vi "MultiQ_09_DataSwitchTimingChanges.vi"() -> ()   [LabVIEW 2021]
doc: "I. Description:\nThis example demonstrates how to acquire a finite amount of data (waveform) using the DAQ device's internal clock.\n\nII. Instructions for Running:\n1. Select the physical channel to correspond to where your signal is input on the DAQ device.\n2. Enter the minimum and maximum voltages.\nNote: For better accuracy try to match the input range to the expected voltage level of the measured signal.\n3. Select the number of samples to acquire.\n4. Set the rate of the acquisition\nNote: The rate should be AT LEAST twice as fast as the maximum frequency component of the signal being acquired.\n\nIII. Block Diagram Steps:\n Steps: \n1. Create an empty task.\n2. Create an analog input voltage channel. Use the DAQmx Base configuration Utility (Tools Menu) to determine the DAQ device name. \n3. Set the rate for the sample clock. Additionally, define the sample mode to be finite and set the number of samples to be acquired per channel.\n4. Call the Start VI to start the acquisition.\n5. Use the Read VI to measure multiple samples from N Channels on the device. Set a timeout so an error is returned if the samples are not returned in the specified time limit\n6. Stop the Analog Input Task.\n7. Call the Clear Task VI to clear the Task.\n8. Use the popup dialog box to display an error if any.\n \nIV. I/O Connections Overview:\nMake sure your signal input terminal matches the Physical Channel I/O Control. For further connection information, refer to your hardware reference manual."
uses:
  <vilib>/Utility/error.llb/DialogType.ctl
  <vilib>/DAQmx/write.llb/DAQmx Write (Analog 2D DBL NChan NSamp).vi
  <vilib>/DAQmx/read.llb/DAQmx Read (Analog 2D DBL NChan NSamp).vi
  <vilib>/measure/maspectr.llb/FFT Power Spectrum and PSD for 1 Chan.vi
  <vilib>/DAQmx/create/channels.llb/DAQmx Create Channel (AI-Voltage-Basic).vi
  <vilib>/DAQmx/configure/timing.llb/DAQmx Timing (Sample Clock).vi
  <vilib>/DAQmx/create/channels.llb/DAQmx Create Channel (AO-Voltage-Basic).vi
  <vilib>/DAQmx/configure/trigger.llb/DAQmx Start Trigger (Digital Edge).vi
  <vilib>/DAQmx/miscellaneous.llb/DAQmx Fill In Error Info.vi
  <vilib>/Analysis/2dsp.llb/Decimate (continuous, DBL).vi
  <vilib>/measure/macond.llb/IIR Filter for 1 Chan.vi
  <vilib>/measure/NI_MAPro.lvlib
  <vilib>/measure/NI_MABase.lvlib
  <vilib>/Analysis/NI_AALPro.lvlib
  <resource>/objmgr/daqmx.rc
panel:
  in  "Run Duration (s) 2":u32=100 caption="Duration (s)"
  out "Nodal Modes":dbl[](array[numeric])=[1092.3, 1649.9, 2505.8]
  out "PlotLabelSize":i32[](array[numeric])
  out "PlotModeSize":i32[](array[numeric])
  out "PlotFreqArray":dbl[][](array[numeric])
  out "PlotLabelArray":string[][](array[string])
  out "Shear Modes":dbl[](array[numeric])=[1092.3, 1649.9, 2505.8]
  out "All Modes":dbl[](array[numeric])=[1092.3, 1649.9, 2505.8]
  out "Modes 10-12":dbl[](array[numeric])=[10072.0, 11259.0, 12454.0]
  out "Modes 7-9":dbl[](array[numeric])=[6683.3, 7225.3, 9346.1]
  in  "Sample Modes":u16(ring)=1 items=["All Modes", "Shear Modes"]
  out "Plot7Label":string="Mode 15: 15961 Hz"
  out "Plot5Label":string="Mode 9: 9346 Hz"
  out "Plot3Label":string="Mode 5: 4361 Hz"
  out "Plot1Label":string="Mode 1: 1092 Hz"
  out "Plot8Label":string="Mode 18: 19859 Hz"
  out "Plot6Label":string="Mode 12: 12454 Hz"
  out "Plot4Label":string="Mode 6: 6645 Hz"
  out "Plot2Label":string="Mode 3: 2506 Hz"
  in  "Ring":u16(ring) items=["EXCITE", "ACQUIRE", "X-Y"]
  in  "Max Value":dbl=10.0 format="%#_13g"
  in  "Min Value":dbl=-10.0 format="%#_13g"
  out "Modes 4-6":dbl[](array[numeric])=[3847.7, 4361.2, 6645.1]
  out "Modes 1-3":dbl[](array[numeric])=[1092.3, 1649.9, 2505.8]
  out "Converted Data Size":i32[](array[numeric])
  out "Raw Data Size":i32[](array[numeric])
  in  "Input Data Type":u16(ring) items=["X Y SUM", "Q 1+/- -- 4+/-", "Q 1-4"]
  in  "Mode Scale":dbl=1.0 min=0.5 max=2.0
  in  "Range (%)":dbl=1.0
  in  "Pressure (t)":sgl=1e-06
  in  "LeverArm (m)":dbl=1.0 min=1.0 max=10000.0
  in  "ADC Range":u16(ring)=6 items=["±0.1 V", "±0.2 V", "±0.5 V", "±1 V", "±2 V", "±5 V", "±10 V"]
  out "PlotLimit":u64
  out "Plot":i32
  in  "Type":u16(ring)=1 items=["Power Spectrum", "PS Density"]
  in  "Unit":u16(ring)=3 items=["Volts", "mRad (full)", "mRad (o2)", "mRad (o1)"]
  in  "Averaging":T1={"Averaging"=enum."No averaging", "weighting mode"=enum."Linear", "number of averages"=10} {"number of averages" min=1 step=1}
  out "Progress":u8(slide) scale=0.0..100.0
  in  "Who":string(combo)="SP"
  in  "fMinPlot":dbl=0.5
  in  "fMaxPlot":dbl=15.0 min=1.0 max=100.0
  in  "Substrate":u16(ring)=1 items=["Silica: 75 x 0.3 mm", "Silica: 75 x 1.0 mm", "Silica: 75 x 2.54 mm"]
  in  "Oversample":bool=TRUE
  in  "fOversample":dbl=50.0 format="%#_13g"
  in  "Span":u32(ring)=60 items=["20 s"=20, "40 s"=40, "1 min"=60, "3 min"=180, "5 min"=300]
  in  "Offset (V)":sgl=2.0
  in  "Ampl. (V)":sgl=2.0
  out "NAve":dbl format="%#_13g"
  out "ADCScale":dbl format="%#_13g"
  out "SizeTimeSeries":i32
  out "BufferPeriod":dbl format="%#_13g"
  out "PSD X":cluster{"f0":dbl, "df":dbl, dbl[][]}(graph)
  out "PlotUnitIndex":u16
  out "DataFilePath":path
  out "fSampleAcquire":dbl format="%#_13g"
  out "NDataPointsOutput":u64
  out "DeltaTOutput":dbl format="%#_13g"
  out "fSampleOutput":dbl format="%#_13g"
  out "DecimFactor":u32
  in  "Comment":string
  out "WriteNumber":i32
  out "WriteLimit":i32
  out "Step":i32
  out "Location":string
  out "PathAtOpen":path
  out "PathAtClose":path
  out "RunLight":bool
  in  "Temp Path":path
  in  "stop":bool
  out "Plot8":cluster{"f0":dbl, "df":dbl, dbl[][]}(graph)
  out "Plot7":cluster{"f0":dbl, "df":dbl, dbl[][]}(graph)
  out "WriteNewHeader":bool
  out "TempFilePath":path
  out "RunPeriod":dbl format="%#_13g"
  out "NDataPointsAcquire":u64
  out "nPlotPerRun":u64
  out "InitialArray":dbl[][](array[numeric])
  out "time vector":dbl[](array[numeric])
  out "ReZero":dbl[][](array[numeric])
  out "df":dbl format="%#_13g"
  out "PlotPeriod":dbl format="%#_13g"
  in  "Run Duration (s)":u32=100 caption="Duration (s)"
  in  "Run Number":i8=1
  in  "∆f (Hz)":u32(ring)=1 items=["1.00"=1, "0.50"=2, "0.25"=4, "0.10"=10]
  in  "Excite":bool
  out "# Elements Response Queue":i32
  out "BufferPeriod ms":u32
  out "# Elements Drive Queue":i32
  out "High Pass IIR filter specs":T2={"Topology"=enum."Butterworth", "Type"=enum."Bandpass", "Order"=7, "Lower Fc"=2000.0, "Upper Fc"=3800.0, "PB Ripple"=0.025, "SB Attenuation"=90.0}
  out "DeltaTAcquire":dbl format="%#_13g"
  out "BufferPoints":u32
  out "PlotPoints":u32
  out "nBufferPerPlot":u32
  out "fMaxPlotHz":dbl format="%#_13g"
  out "fMinPlotHz":dbl format="%#_13g"
  out "Plot6":cluster{"f0":dbl, "df":dbl, dbl[][]}(graph)
  out "Plot5":cluster{"f0":dbl, "df":dbl, dbl[][]}(graph)
  out "Plot4":cluster{"f0":dbl, "df":dbl, dbl[][]}(graph)
  out "Plot3":cluster{"f0":dbl, "df":dbl, dbl[][]}(graph)
  out "Plot2":cluster{"f0":dbl, "df":dbl, dbl[][]}(graph)
  out "Plot1":cluster{"f0":dbl, "df":dbl, dbl[][]}(graph)
  in  "Start":bool
  out "PSD Y":cluster{"f0":dbl, "df":dbl, dbl[][]}(graph) caption="Measurement"
  out "File":string
  in  "Path":path caption="File Name"
  in  "Label":string
  in  "Name":string
  out "HTML \nTitle":string
  out "Start Time":timestamp
  out "Write Light":bool
  in  "AutoSave":bool=TRUE
  in  "Manual Save":bool=TRUE caption="Saving Data"
  out "Out":path caption="File Name Out"
  in  "QUIT":bool
  # "Acquire"
  # "Multi Q\nVer 0.9.5.0 • July 2021\nSteve Penn"
  # "Sample"
  # "Comment"
  # "Frequency"
  # "kHz"
  # ":"
  # "Oversample"
  # "kHz"
  # "PLOT:"
  # "Mode Plots:"
  # "PSD Y / Excitation"
  # "/"
  # "Averaging"
  # "Drive"
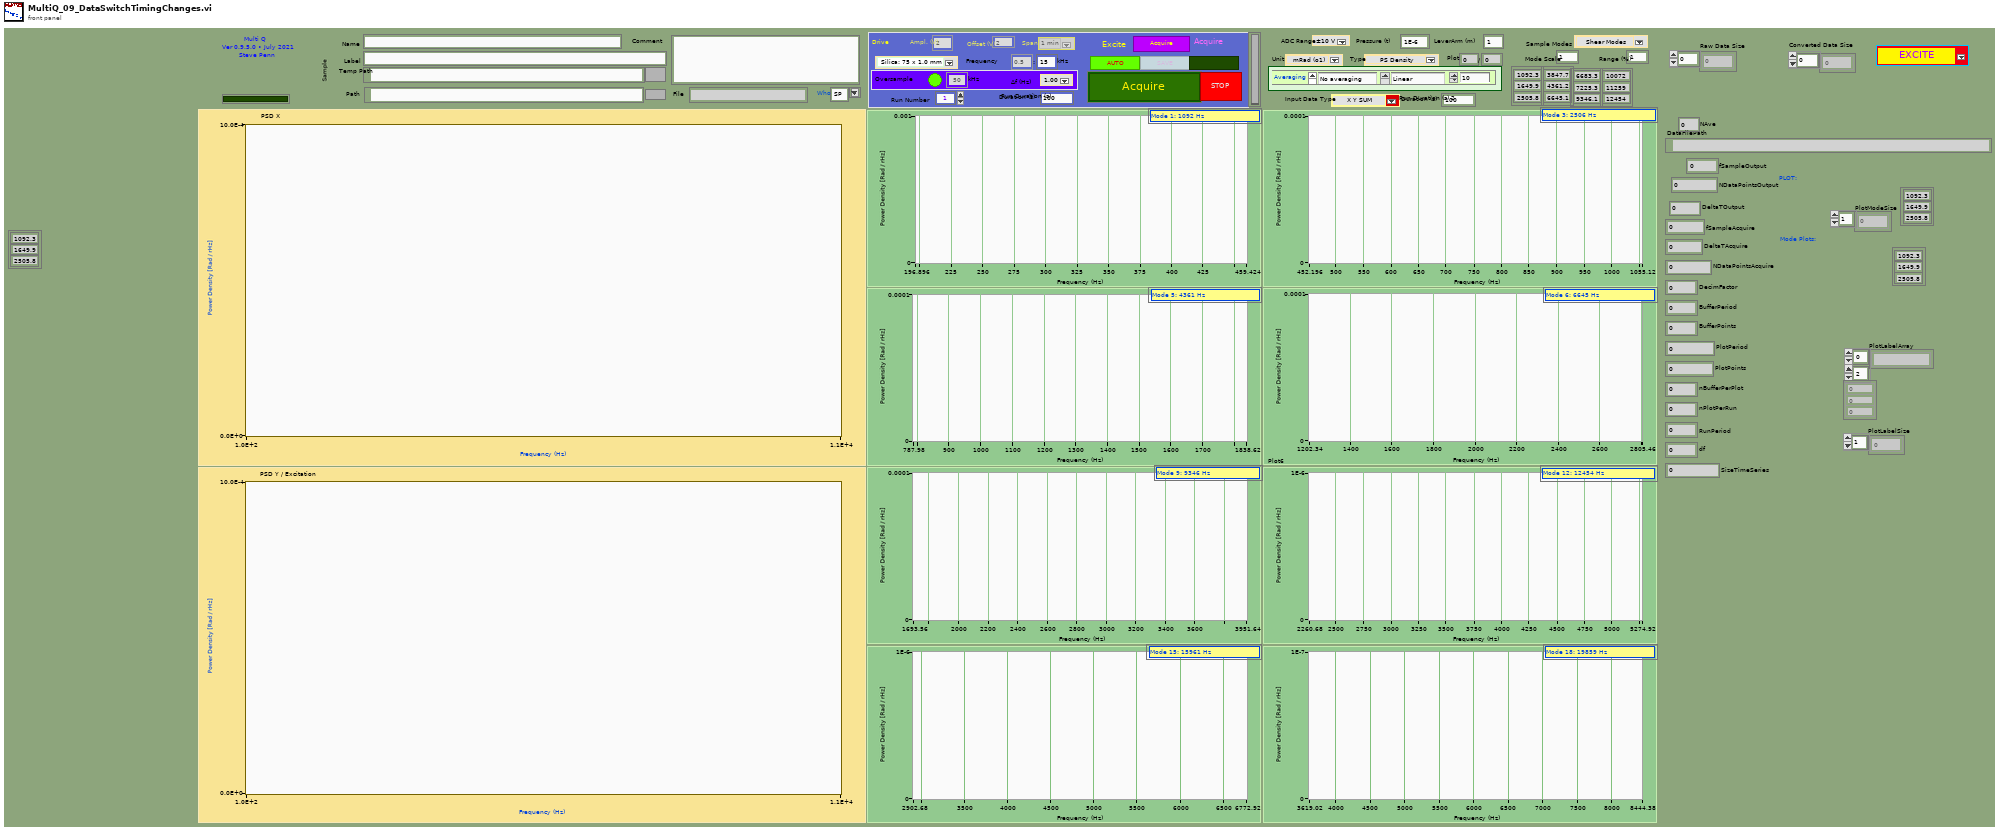
[diagram p1: front panel]
types:
  T1 = cluster{"Averaging":enum16{"No averaging", "Vector averaging", "RMS averaging", "Peak hold"}, "weighting mode":enum16{"Linear", "Exponential"}, "number of averages":u32}
  T2 = cluster{"Topology":enum16{"Off", "Butterworth", "Chebyshev", "Inverse Chebyshev", "Elliptic", "Bessel"}, "Type":enum16{"Lowpass", "Highpass", "Bandpass", "Bandstop"}, "Order":i32, "Lower Fc":dbl, "Upper Fc":dbl, "PB Ripple":dbl, "SB Attenuation":dbl}
  T3 = enum16{"Off", "Butterworth", "Chebyshev", "Inverse Chebyshev", "Elliptic", "Bessel"}
  T4 = enum16{"Lowpass", "Highpass", "Bandpass", "Bandstop"}
  T5 = enum8{"open", "replace", "create", "open or create", "replace or create", "replace or create with confirmation"}
  T6 = enum16{"No averaging", "Vector averaging", "RMS averaging", "Peak hold"}
  T7 = cluster{"Averaging":enum16{"No averaging", "Vector averaging", "RMS averaging", "Peak hold"}, "weighting mode":enum16{"Linear", "Exponential"}, "weighting mode":u64}
  T8 = typedef "DialogType.ctl" = u16
  T9 = enum16{"Left Button", "Center Button", "Right Button", "Window Close"}
  T10 = cluster{"Averaging":enum16{"No averaging", "Vector averaging", "RMS averaging", "Peak hold"}, "weighting mode":enum16{"Linear", "Exponential"}, "Value":u64}
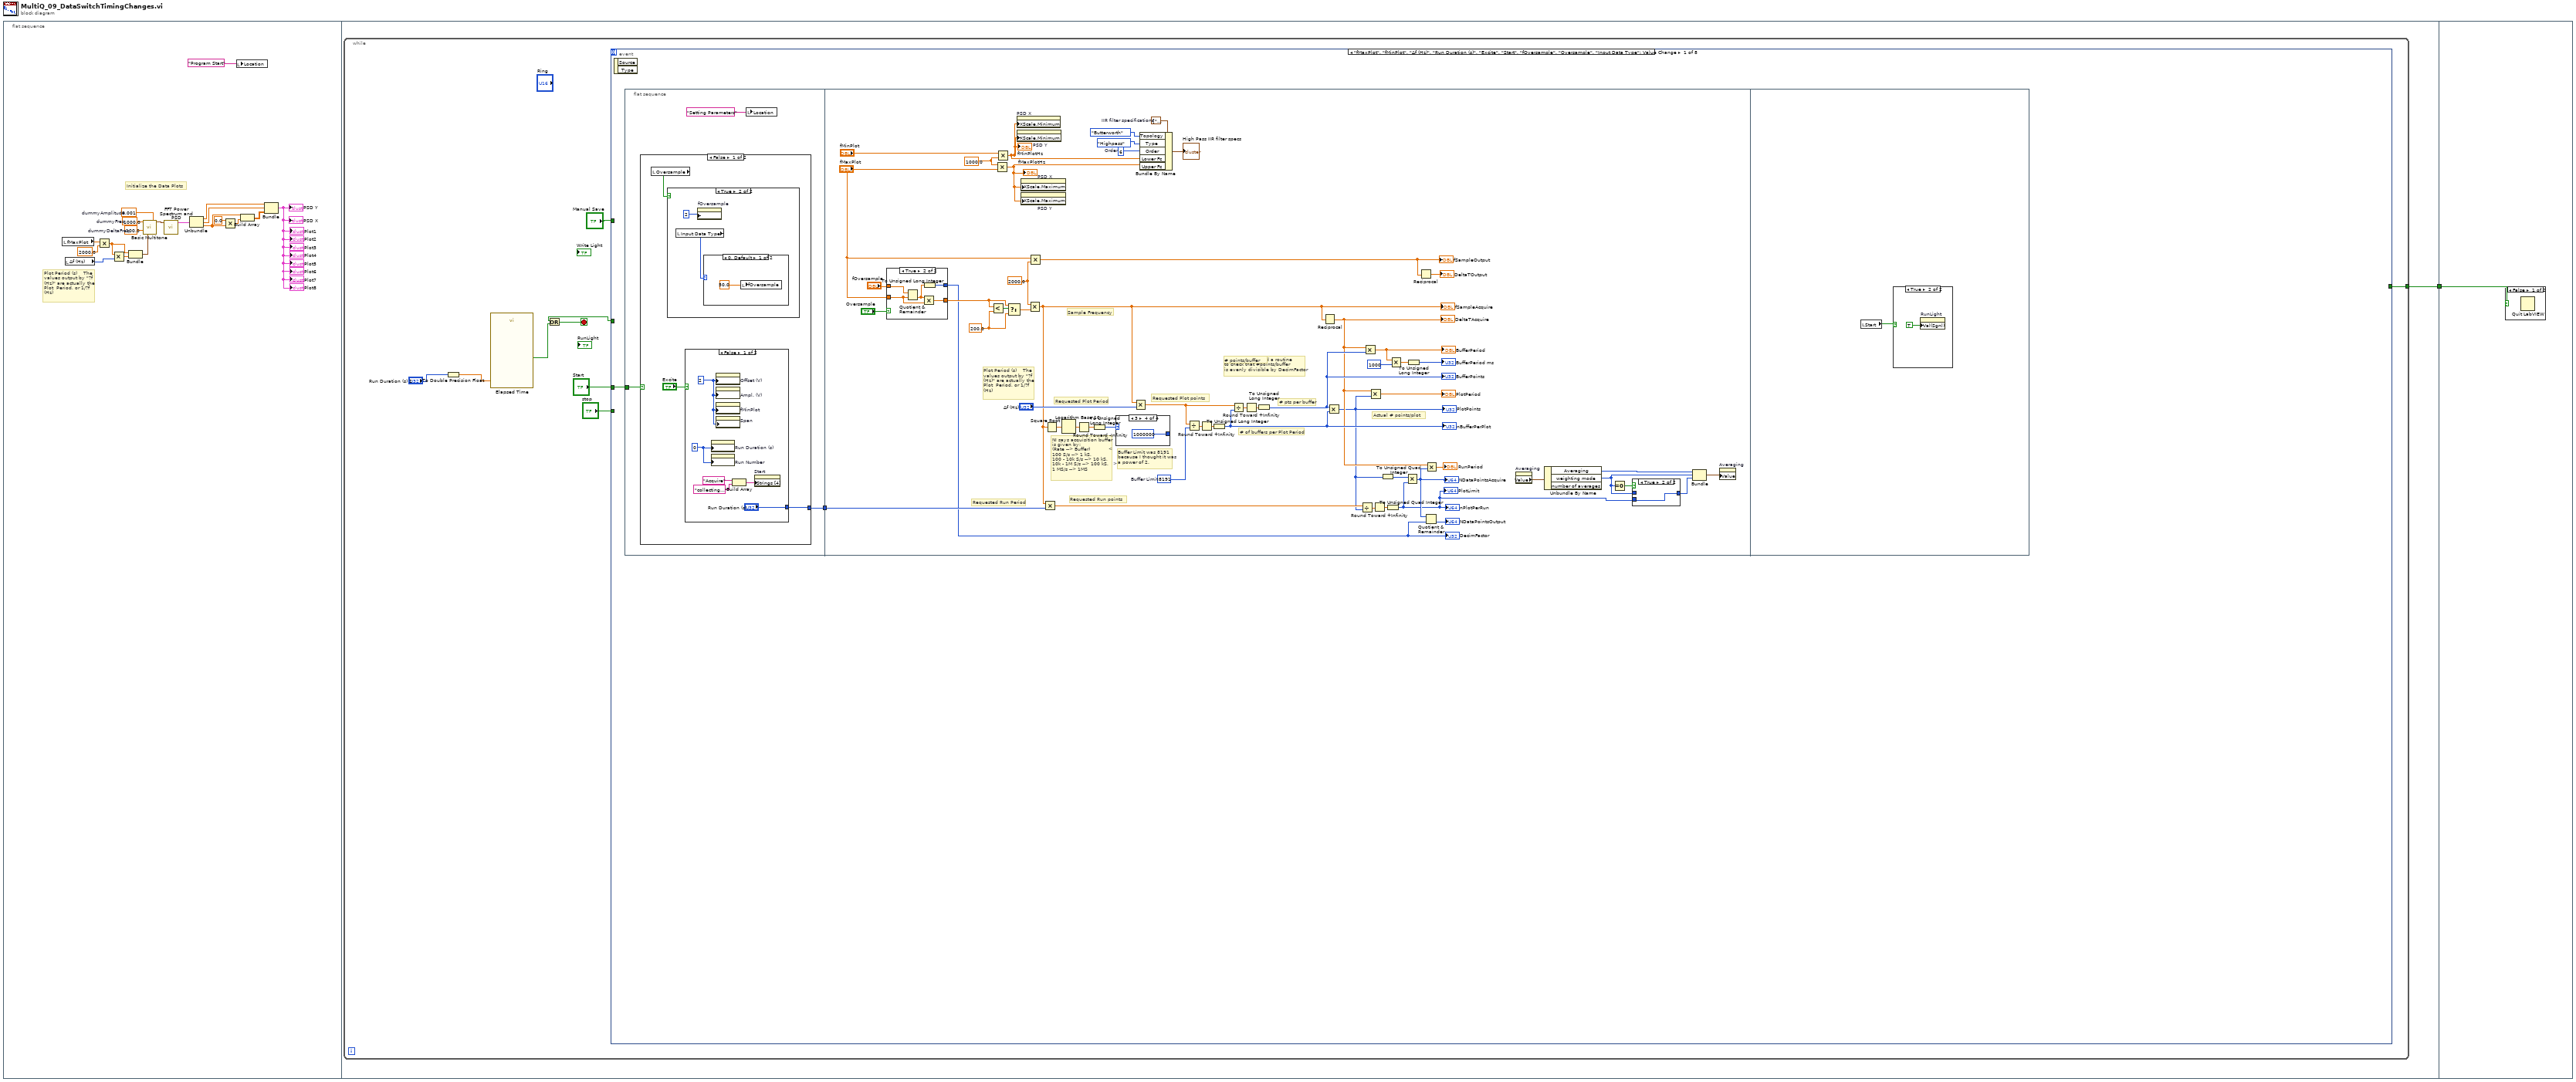
[diagram p0: block diagram]
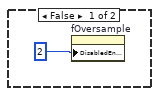
[diagram p2: hidden frame]
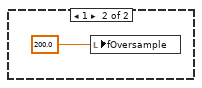
[diagram p3: hidden frame]
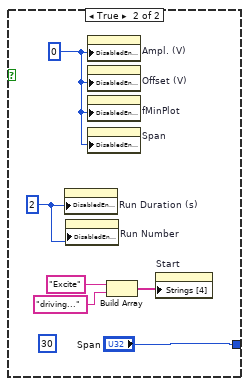
[diagram p4: hidden frame]
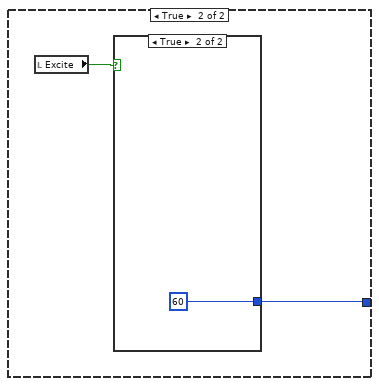
[diagram p5: hidden frame]
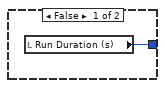
[diagram p6: hidden frame]
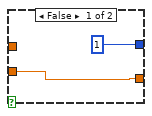
[diagram p8: hidden frame]
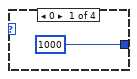
[diagram p9: hidden frame]
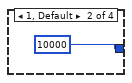
[diagram p10: hidden frame]
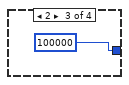
[diagram p11: hidden frame]
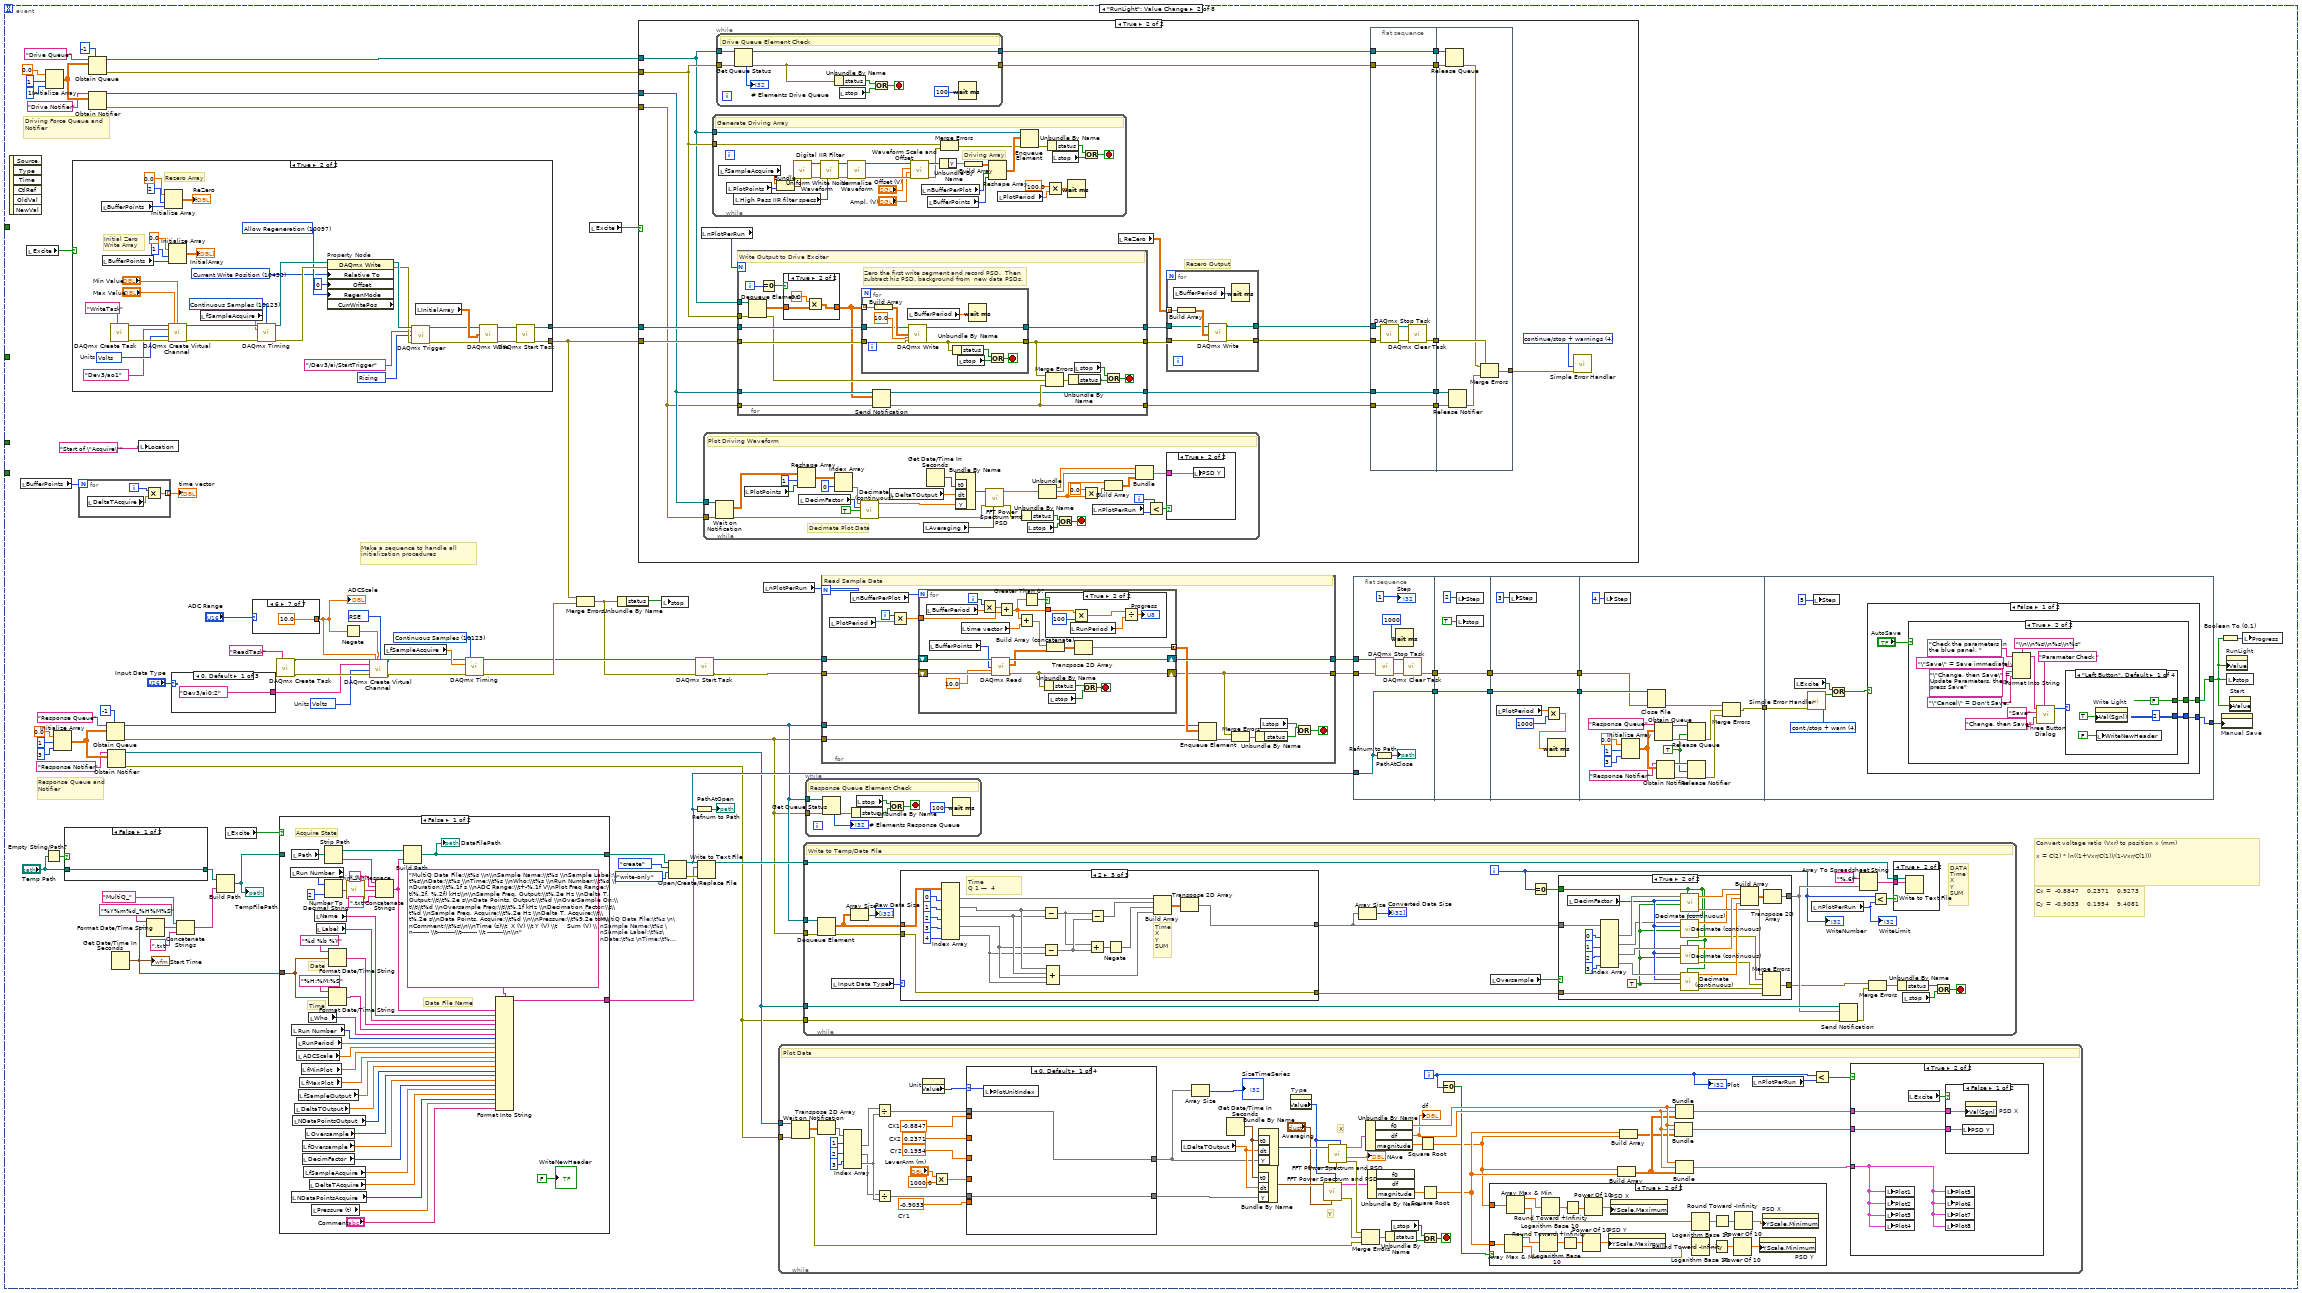
[diagram p13: hidden frame]
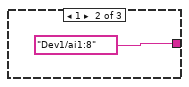
[diagram p14: hidden frame]
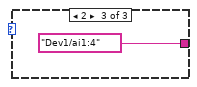
[diagram p15: hidden frame]
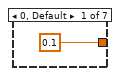
[diagram p16: hidden frame]
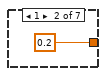
[diagram p17: hidden frame]
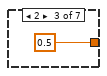
[diagram p18: hidden frame]
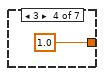
[diagram p19: hidden frame]
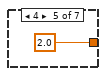
[diagram p20: hidden frame]
diagram:
  n1 = flat-sequence {
    tunnel: [w21] -> w1
    tunnel: w1 -> [w1123]
    frame #0 {
      w4 = 0.001  # dummyAmplitude
      w2 = 100.0  # dummyDeltaFreq
      w3 = 1000.0  # dummyFreq
      # "Initialize the Data Plots"
      # "Plot Period (s)    The values output by \"?f (Hz)\" are actually the Plot  Period, or 1/?f (Hz)"
      n2 = local read "fMaxPlot"() -> (w9:dbl)
      n3 = local read "∆f (Hz)"() -> (w8:u32)
      n4 = Multiply(x=w9, y=2000.0) -> (x*y=w6:dbl)
      n5 = Multiply(x=w6, y=w8) -> (x*y=w7:dbl)
      n6 = Bundle(w6, w7) -> (w19:cluster{dbl, dbl})  [unwired: 1 in]
      n7 = call <vilib>:"Basic Multitone.vi"("start frequency"=w3, "amplitude"=w4, "delta frequency"=w2, "sampling info"=w19) -> ("signal out"=w18:waveform(dbl))  [unwired: 8 in, 3 out]
      n8 = call-poly <vilib>:"FFT Power Spectrum and PSD.vi"("time signal"=w18) -> ("Power Spectrum / PSD"=w11:cluster{"f0":dbl, "df":dbl, "magnitude":dbl[]})  [unwired: 7 in, 3 out]
      n9 = Unbundle(w11) -> ("f0"=w16:dbl, "df"=w13:dbl, "magnitude"=w12:dbl[])
      n10 = Multiply(x=0.0, y=w12) -> (x*y=w14:dbl[])
      n11 = local write "Location"("Program Start") -> ()
      n12 = Build Array(w12, w14) -> (w15:dbl[][])
      n13 = Bundle("f0"=w16, "df"=w13, w15) -> (→"PSD Y" →"PSD X" →"Plot5" →"Plot6" →"Plot7" →"Plot8" →"Plot3" →"Plot1" →"Plot2" →"Plot4":cluster{"f0":dbl, "df":dbl, dbl[][]})  [unwired: 1 in]
    }
    frame #1 {
      n14 = while {
        tunnel: [w30] -> w21
        stop <- w22 stop-if-true
        n15 = To Double Precision Float(number="Run Duration (s) 2") -> (double precision float=w25:dbl)
        n16 = call "Elapsed Time"("Time Target (s)"=w25) -> ("Time has Elapsed"=w24:bool)  [unwired: 11 in, 7 out]
        n17 = event shown="[0] \"fMaxPlot\", \"fMinPlot\", \"∆f (Hz)\", \"Run Duration (s)\", \"Excite\", \"Start\", \"fOversample\", \"Oversample\", \"Input Data Type\": Value Change" {
          selector: _ -> [_ _ _ _ _ _ _ _]
          dyn-events: _ -> [_ _ _ _ _ _ _ _]
          timeout: _ -> [_ _ _ _ _ _ _ _]
          tunnel: [_ _ _ _ _ _ w1098 _] -> w23
          tunnel: [_ _ _ _ _ _ w1099 _] -> w30
          tunnel: "Manual Save" -> [_ _ _ _ _ _ _ _]
          tunnel: "Start" -> [w31 _ _ _ _ _ _ _]
          tunnel: "stop" -> [_ _ _ _ _ _ _ _]
          event "fMaxPlot", "fMinPlot", "∆f (Hz)", "Run Duration (s)", "Excite", "Start", "fOversample", "Oversample", "Input Data Type": Value Change {
            n18 = event-data() -> ()  [unwired: 3 out]
            n19 = flat-sequence {
              tunnel: [w35] -> w32
              tunnel: w31 -> [w34]
              tunnel: w32 -> [w81]
              frame #0 {
                n20 = case shown="False" w34 {
                  tunnel: [w37 w56] -> w35
                  frame False {
                    n21 = local read "Oversample"() -> (w36:bool)
                    n22 = case shown="True" w36 {
                      frame False {
                        n23 = property on="fOversample" class="DigNum (strict)"("DisabledEnum"=2) -> ()  [unwired: 2 in, 2 out]
                      }
                      frame True {
                        n24 = local read "Input Data Type"() -> (w40:u16)
                        n25 = property on="fOversample" class="DigNum (strict)"("DisabledEnum"=2) -> ()  [unwired: 2 in, 2 out]
                        n26 = case shown="0, Default" w40 {
                          frame 0, Default {
                            n27 = local write "fOversample"(50.0) -> ()
                          }
                          frame 1 {
                            n28 = local write "fOversample"(200.0) -> ()
                          }
                        }
                      }
                    }
                    n29 = case shown="False" "Excite" {
                      tunnel: ["Run Duration (s)" "Span"] -> w37
                      frame False {
                        w46 = 0
                        w44 = 2
                        n30 = property on="Run Duration (s)" class="DigNum (strict)"("DisabledEnum"=w46) -> ()  [unwired: 2 in, 2 out]
                        n31 = property on="Run Number" class="DigNum (strict)"("DisabledEnum"=w46) -> ()  [unwired: 2 in, 2 out]
                        n32 = property on="Offset (V)" class="DigNum (strict)"("DisabledEnum"=w44) -> ()  [unwired: 2 in, 2 out]
                        n33 = property on="Ampl. (V)" class="DigNum (strict)"("DisabledEnum"=w44) -> ()  [unwired: 2 in, 2 out]
                        n34 = property on="fMinPlot" class="DigNum (strict)"("DisabledEnum"=w44) -> ()  [unwired: 2 in, 2 out]
                        n35 = property on="Span" class="Ring (strict)"("DisabledEnum"=w44) -> ()  [unwired: 2 in, 2 out]
                        n36 = Build Array("Acquire", "collecting...") -> (w49:string[])
                        n37 = property on="Start" class="Bool (strict)"("Strings [4]"=w49) -> ()  [unwired: 2 in, 2 out]
                      }
                      frame True {
                        (unwired) 30
                        w52 = 2
                        w51 = 0
                        n38 = property on="Run Duration (s)" class="DigNum (strict)"("DisabledEnum"=w52) -> ()  [unwired: 2 in, 2 out]
                        n39 = property on="Run Number" class="DigNum (strict)"("DisabledEnum"=w52) -> ()  [unwired: 2 in, 2 out]
                        n40 = property on="Ampl. (V)" class="DigNum (strict)"("DisabledEnum"=w51) -> ()  [unwired: 2 in, 2 out]
                        n41 = property on="Offset (V)" class="DigNum (strict)"("DisabledEnum"=w51) -> ()  [unwired: 2 in, 2 out]
                        n42 = property on="fMinPlot" class="DigNum (strict)"("DisabledEnum"=w51) -> ()  [unwired: 2 in, 2 out]
                        n43 = property on="Span" class="Ring (strict)"("DisabledEnum"=w51) -> ()  [unwired: 2 in, 2 out]
                        n44 = Build Array("Excite", "driving...") -> (w55:string[])
                        n45 = property on="Start" class="Bool (strict)"("Strings [4]"=w55) -> ()  [unwired: 2 in, 2 out]
                      }
                    }
                  }
                  frame True {
                    n46 = local read "Excite"() -> (w57:bool)
                    n47 = case shown="True" w57 {
                      tunnel: [w58 60] -> w56
                      frame False {
                        n48 = local read "Run Duration (s)"() -> (w58:u32)
                      }
                      frame True {
                      }
                    }
                  }
                }
                n49 = local write "Location"("Setting Parameters") -> ()
              }
              frame #1 {
                w102 = 6  # Order
                w105 = T2 {"Topology"=enum."Butterworth", "Type"=enum."Bandpass", "Order"=7, "Lower Fc"=2000.0, "Upper Fc"=3800.0, "PB Ripple"=0.025, "SB Attenuation"=90.0}  # IIR filter specifications
                w111 = 1000.0
                w91 = 8191  # Buffer Limit
                w78 = 2000.0
                w110 = 200.0
                # "# pts per buffer"
                # "I may need to add a routine \nto check that #points/buffer\nis evenly divisible by DecimFactor"
                # "Requested Run points"
                # "Requested Run Period"
                # "Requested Plot Period"
                # "NI says acquisition buffer  is given by:                   (Rate --> Buffer)            < 100 S/s --> 1 kS,                 100 - 10k S/s --> 10 kS,   10k - 1M S/s --> 100 kS,   > 1 MS/s --> 1MS"
                # "Buffer Limit was 8191 because I thought it was a power of 2."
                # "Plot Period (s)    The values output by \"?f (Hz)\" are actually the Plot  Period, or 1/?f (Hz)"
                # "Sample Frequency"
                # "Actual # points/plot"
                # "# points/buffer"
                # "Requested Plot points"
                # "# of buffers per Plot Period"
                n50 = case shown="True" "Oversample" {
                  tunnel: "fOversample" -> [_ w124]
                  tunnel: [w119 w123] -> w79
                  tunnel: "fMaxPlot" -> [w119 w122]
                  tunnel: [1 w121] -> w71
                  frame False {
                  }
                  frame True {
                    n51 = Quotient & Remainder(x=w124, y=w122) -> (floor(x/y)=w120:dbl)  [unwired: 1 out]
                    n52 = Multiply(x=w120, y=w122) -> (x*y=w123:dbl)
                    n53 = To Unsigned Long Integer(number=w120) -> (unsigned 32bit integer=w121:u32)
                  }
                }
                "DecimFactor" <- w71
                n54 = Less?(x=w79, y=w110) -> (x < y?=w115:bool)
                n55 = Multiply(x=w111, y="fMaxPlot") -> (x*y=w69:dbl)
                "fMaxPlotHz" <- w69
                n56 = Multiply(x="fMinPlot", y=w111) -> (x*y=w70:dbl)
                "fMinPlotHz" <- w70
                n57 = Select(t=w79, s=w115, f=w110) -> (s? t:f=w114:dbl)
                n58 = property on="PSD X" class="WFGraph (strict)"("XScale.Minimum"=w70) -> ()  [unwired: 2 in, 2 out]
                n59 = property on="PSD Y" class="WFGraph (strict)"("XScale.Minimum"=w70) -> ()  [unwired: 2 in, 2 out]
                n60 = property on="PSD X" class="WFGraph (strict)"("XScale.Maximum"=w69) -> ()  [unwired: 2 in, 2 out]
                n61 = property on="PSD Y" class="WFGraph (strict)"("XScale.Maximum"=w69) -> ()  [unwired: 2 in, 2 out]
                n62 = Multiply(x=w78, y=w114) -> (x*y=w88:dbl)
                "fSampleAcquire" <- w88
                n63 = Multiply(x="fMaxPlot", y=w78) -> (x*y=w76:dbl)
                "fSampleOutput" <- w76
                n64 = Multiply(x=w88, y=w81) -> (x*y=w87:dbl)
                n65 = Square Root(x=w88) -> (sqrt(x)=w96:dbl)
                n66 = Logarithm Base 10(1:w96) -> (0:w95:dbl)
                n67 = Round Toward -Infinity(1:w95) -> (0:w94:dbl)
                n68 = To Unsigned Long Integer(number=w94) -> (unsigned 32bit integer=w93:u32)
                n69 = case shown="3" w93 {
                  tunnel: [1000 10000 100000 1000000] -> _
                  frame 0 {
                  }
                  frame 1, Default {
                  }
                  frame 2 {
                  }
                  frame 3 {
                  }
                }
                n70 = Multiply(x=w88, y="∆f (Hz)") -> (x*y=w113:dbl)
                n71 = Bundle By Name(cluster=w105, "Topology"=T3."Butterworth", "Type"=T4."Highpass" ("Enum"), "Order"=w102, "Lower Fc"=w70, "Upper Fc"=w69) -> (→"High Pass IIR filter specs":T2)
                n72 = Divide(x=w113, y=w91) -> (x/y=w109:dbl)
                n73 = Round Toward +Infinity(x=w109) -> (ceil(x): smallest int >= x=w108:dbl)
                n74 = To Unsigned Long Integer(number=w108) -> (unsigned 32bit integer=w106:u32)
                "nBufferPerPlot" <- w106
                n75 = Divide(x=w113, y=w106) -> (x/y=w112:dbl)
                n76 = Round Toward +Infinity(x=w112) -> (ceil(x): smallest int >= x=w107:dbl)
                n77 = To Unsigned Long Integer(number=w107) -> (unsigned 32bit integer=w84:u32)
                "BufferPoints" <- w84
                n78 = Reciprocal(x=w88) -> (1/x=w83:dbl)
                "DeltaTAcquire" <- w83
                n79 = Multiply(x=w84, y=w106) -> (x*y=w60:u32)
                "PlotPoints" <- w60
                n80 = Divide(x=w87, y=w60) -> (x/y=w86:dbl)
                n81 = Multiply(x=w83, y=w84) -> (x*y=w99:dbl)
                "BufferPeriod" <- w99
                n82 = Multiply(x=w83, y=w60) -> (x*y=→"PlotPeriod":dbl)
                n83 = Round Toward +Infinity(x=w86) -> (ceil(x): smallest int >= x=w85:dbl)
                n84 = To Unsigned Quad Integer(1:w60) -> (0:w61:u64)
                n85 = To Unsigned Quad Integer(1:w85) -> (0:w62:u64)
                "nPlotPerRun" <- w62
                "PlotLimit" <- w62
                n86 = Multiply(x=w99, y=1000) -> (x*y=w98:dbl)
                n87 = Multiply(x=w61, y=w62) -> (x*y=w74:u64)
                "NDataPointsAcquire" <- w74
                n88 = To Unsigned Long Integer(number=w98) -> (unsigned 32bit integer=→"BufferPeriod ms":u32)
                n89 = Reciprocal(x=w76) -> (1/x=→"DeltaTOutput":dbl)
                n90 = Quotient & Remainder(x=w74, y=w71) -> (floor(x/y)=→"NDataPointsOutput":u64)  [unwired: 1 out]
                n91 = Multiply(x=w83, y=w74) -> (x*y=→"RunPeriod":dbl)
                n92 = property on="Averaging" class="Clust (strict)"() -> ("Value"=w64:T1)  [unwired: 2 in, 2 out]
                n93 = Unbundle By Name(w64) -> ("Averaging"=w65:T6, "weighting mode"=w68:enum16{"Linear", "Exponential"})  [unwired: 1 out]
                n94 = Equal To 0?(x=w68) -> (x = 0?=w66:bool)
                n95 = case shown="True" w66 {
                  tunnel: [w116 w117] -> w67
                  tunnel: w68 -> [w116 _]
                  tunnel: w62 -> [_ w117]
                  frame False {
                  }
                  frame True {
                  }
                }
                n96 = Bundle("Averaging"=w65, "weighting mode"=w68, "weighting mode"=w67) -> (w63:T7)  [unwired: 1 in]
                n97 = property on="Averaging" class="Clust (strict)"("Value"=w63) -> ()  [unwired: 2 in, 2 out]
              }
              frame #2 {
                n98 = local read "Start"() -> (w129:bool)
                n99 = case shown="True" w129 {
                  frame False {
                  }
                  frame True {
                    n100 = property on="RunLight" class="Bool (strict)"("Val(Sgnl)"=TRUE) -> ()  [unwired: 2 in, 2 out]
                  }
                }
              }
            }
          }
          event "RunLight": Value Change {
            w139 = 10123 items=["Finite Samples"=10178, "Continuous Samples"=10123] ("sample mode")
            w141 = 10348 items=["Volts"=10348]  # Units
            w146 = 10083 items=["default"=-1, "differential"=10106, "RSE"=10083, "NRSE"=10078] ("input terminal configuration")
            # "Cx =  -0.8847    0.2371    0.9273\n\nCy =  -0.9033    0.1954    9.4081"
            # "Convert voltage ratio (Vxr) to position x (mm)\n\nx = C(2) * ln((1+Vxr/C(1))/(1-Vxr/C(1)))"
            # "Response Queue and Notifier"
            # "Driving Force Queue and Notifier"
            # "Make a sequence to handle all initialization procedures"
            n101 = event-data() -> ()  [unwired: 7 out]
            n102 = local read "BufferPoints"() -> (w202:u32)
            n103 = local read "Excite"() -> (w199:bool)
            n104 = Empty String/Path?(string/path="Temp Path") -> (empty?=w187:bool)
            n105 = Initialize Array(0.0, 1, 1) -> (w176:dbl[][])
            n106 = Initialize Array(0.0, 1, 3) -> (w165:dbl[][])
            n107 = case shown="False" w187 {
              tunnel: "Temp Path" -> [w480 _]
              tunnel: [w480 w481] -> w185
              frame False {
              }
              frame True {
                w481 = path "/Users/qlab/Documents/MultiQ/Temp"
                n108 = local write "Temp Path"(w481) -> ()
              }
            }
            n109 = case shown="True" w199 {
              tunnel: [w687 w694] -> w198
              tunnel: [w688 w695] -> w200
              frame False {
                n110 = call <vilib>:"DAQmx Create Task.vi"() -> ("task out"=w688:refnum<k21>, "error out"=w687:errorcluster)  [unwired: 14 in]
              }
              frame True {
                w690 = 10430 items=["First Sample"=10424, "Current Write Position"=10430] ("RelativeTo")
                w703 = 10097 items=["Allow Regeneration"=10097, "Do Not Allow Regeneration"=10158] ("RegenMode")
                w699 = 10280 items=["Falling"=10171, "Rising"=10280]
                w706 = 10123 items=["Finite Samples"=10178, "Continuous Samples"=10123] ("sample mode")
                w710 = 10348 items=["Volts"=10348]  # Units
                # "Initial Zero Write Array"
                # "Rezero Array"
                n111 = local read "BufferPoints"() -> (w721:u32)
                n112 = local read "BufferPoints"() -> (w719:u32)
                n113 = call <vilib>:"DAQmx Create Task.vi"("new task name"="WriteTask") -> ("task out"=w712:refnum<k21>, "error out"=w711:errorcluster)  [unwired: 13 in]
                n114 = Initialize Array(0.0, 2, w721) -> (→"ReZero":dbl[][])
                n115 = Initialize Array(0.0, 1, w719) -> (→"InitialArray":dbl[][])
                n116 = call-poly <vilib>:"DAQmx Create Virtual Channel.vi"("task in"=w712, "maximum value"="Max Value", "minimum value"="Min Value", "physical channels"=tag "Dev3/ao1", "units"=w710, "error in"=w711) -> ("task out"=w709:refnum<k21>, "error out"=w708:errorcluster)  [unwired: 8 in]
                n117 = local read "fSampleAcquire"() -> (w707:dbl)
                n118 = call-poly <vilib>:"DAQmx Timing.vi"("task/channels in"=w709, "sample mode"=w706, "rate"=w707, "error in"=w708) -> ("task out"=w705:refnum<k21>, "error out"=w704:errorcluster)  [unwired: 10 in]
                n119 = property on="Property Node" class="DAQmx Write" props=["Relative To", "Offset", "RegenMode", "CurrWritePos"](reference=w705, error in=w704, "Relative To"=w690, "Offset"=0, "RegenMode"=w703) -> (reference out=w702:refnum<k21>, error out=w701:errorcluster)  [unwired: 1 out]
                n120 = call-poly <vilib>:"DAQmx Trigger.vi"("task/channels in"=w702, "source"=tag "/Dev3/ai/StartTrigger" ("DAQmx Terminal"), "edge"=w699, "error in"=w701) -> ("task out"=w697:refnum<k21>, "error out"=w696:errorcluster)  [unwired: 10 in]
                n121 = local read "InitialArray"() -> (w698:dbl[][])
                n122 = call-poly <vilib>:"DAQmx Write.vi"("task/channels in"=w697, "data"=w698, "error in"=w696) -> ("task out"=w692:refnum<k21>, "error out"=w693:errorcluster)  [unwired: 10 in, 1 out]
                n123 = call <vilib>:"DAQmx Start Task.vi"("task/channels in"=w692, "error in"=w693) -> ("task out"=w695:refnum<k21>, "error out"=w694:errorcluster)  [unwired: 12 in]
              }
            }
            n124 = for {
              N: w202 -> [_]
              tunnel: [w811] -> w201 mode=indexing
              i -> [w809]
              n125 = local read "DeltaTAcquire"() -> (w810:dbl)
              n126 = Multiply(x=w809, y=w810) -> (x*y=w811:dbl)
            }
            "time vector" <- w201
            n127 = Obtain Queue(max queue size (-1, unlimited)=-1, name (unnamed)="Drive Queue", element data type=w176) -> (queue out=w167:refnum<queue>, error out=w166:errorcluster)  [unwired: 2 in, 1 out]
            n128 = Obtain Notifier(name (unnamed)="Drive Notifier", notification data type=w176) -> (notifier out=w169:refnum<notifier>, error out=w168:errorcluster)  [unwired: 2 in, 1 out]
            n129 = Obtain Queue(max queue size (-1, unlimited)=-1, name (unnamed)="Response Queue", element data type=w165) -> (queue out=w157:refnum<queue>, error out=w156:errorcluster)  [unwired: 2 in, 1 out]
            n130 = Obtain Notifier(name (unnamed)="Response Notifier", notification data type=w165) -> (notifier out=w155:refnum<notifier>, error out=w154:errorcluster)  [unwired: 2 in, 1 out]
            n131 = Get Date/Time In Seconds() -> (seconds since 1Jan1904=w184:timestamp)
            "Start Time" <- w184
            n132 = local write "Location"("Start of \"Acquire\"") -> ()
            n133 = Format Date/Time String(time format string (%c)="%Y%m%d_%H%M%S", seconds (now)=w184) -> (date/time string=w210:string)  [unwired: 1 in]
            n134 = case shown="0, Default" "Input Data Type" {
              tunnel: [tag "Dev3/ai0:2" ("DAQmx Physical Channel") tag "Dev1/ai1:8" ("DAQmx Physical Channel") tag "Dev1/ai1:4" ("DAQmx Physical Channel")] -> w140
              frame 0, Default {
              }
              frame 1 {
              }
              frame 2 {
              }
            }
            n135 = Concatenate Strings("MultiQ_", w210, ".txt") -> (w189:string)
            n136 = Build Path(base path=w185, name or relative path=w189) -> (appended path=w188:path)
            "TempFilePath" <- w188
            n137 = local read "Excite"() -> (w196:bool)
            n138 = case shown="6" "ADC Range" {
              tunnel: [0.1 ("Max Value") 0.2 ("Max Value") 0.5 ("Max Value") 1.0 ("Max Value") 2.0 ("Max Value") 5.0 ("Max Value") 10.0 ("Max Value")] -> w145
              frame 0, Default {
              }
              frame 1 {
              }
              frame 2 {
              }
              frame 3 {
              }
              frame 4 {
              }
              frame 5 {
              }
              frame 6 {
              }
            }
            "ADCScale" <- w145
            n139 = call <vilib>:"DAQmx Create Task.vi"("new task name"="ReadTask") -> ("task out"=w143:refnum<k21>, "error out"=w142:errorcluster)  [unwired: 13 in]
            n140 = case shown="False" w196 {
              tunnel: [w499 w523] -> w205
              tunnel: w184 -> [w508 w522]
              tunnel: [w498 w521] -> w195
              tunnel: w188 -> [_ w521]
              frame False {
                w507 = "MultiQ Data File:\\t%s \\n\\nSample Name:\\t%s \\nSample Label:\\t%s\\nDate:\\t%s \\nTime:\\t%s \\nWho:\\t%s \\nRun Number:\\t%d \\nDuration:\\t%.1f s \\nADC Range:\\t+-%.1f V\\nPlot Freq Range:\\t(%.2f, %.2f) kHz\\n\\nSample Freq, Output:\\t%.2e Hz \\nDelta T, Output:\\t\\t%.2e s\\nData Points, Output:\\t%d \\nOverSample On:\\t\\t\\t%d \\nOversample Freq:\\t\\t%.1f kHz \\nDecimation Factor:\\t\\t%d \\nSample Freq, Acquire:\\t%.2e Hz \\nDelta T, Acquire:\\t\\t%.2e s\\nData Points, Acquire:\\t%d \\n\\nPressure:\\t%9.2e torr\\nComment:\\t%s\\n\\nTime (s)\\t  X (V) \\t Y (V) \\t     Sum (V) \\n-------- \\t---------\\t-------- \\t --------\\n\\n"  # MultiQ Data File:\t%s \n\nSample Name:\t%s \nSample Label:\t%s\nDate:\t%s \nTime:\t%s \nWho:\t%s \nRun Number:\t%d \nDuration:\t%.1f s \nADC Range:\t+-%.1f V\nPlot Freq Range:\t(%.2f, %.2f) kHz\n\nSample Freq, Output:\t%.2e Hz \nDelta T, Output:\t\t%.2e s\nData Points, Output:\t%d \nOverSample On:\t\t\t%d \nOversample Freq:\t\t%.1f kHz \nDecimation Factor:\t\t%d \nSample Freq, Acquire:\t%.2e Hz \nDelta T, Acquire:\t\t%.2e s\nData Points, Acquire:\t%d \n\nPressure:\t%9.2e torr\nComment:\t%s\n\nTime (s)\t  X (V) \t Y (V) \t     Sum (V) \n-------- \t---------\t-------- \t --------\n\n
                # "Data File Name"
                # "Date"
                # "Time"
                # "Acquire State"
                n141 = local read "Run Number"() -> (w512:i8)
                n142 = local read "NDataPointsAcquire"() -> (w484:u64)
                n143 = local read "Path"() -> (w511:path)
                n144 = local read "Run Number"() -> (w506:i8)
                n145 = local read "NDataPointsOutput"() -> (w491:u64)
                n146 = local read "DeltaTOutput"() -> (w490:dbl)
                n147 = local read "RunPeriod"() -> (w500:dbl)
                n148 = local read "ADCScale"() -> (w495:dbl)
                n149 = local read "fSampleOutput"() -> (w492:dbl)
                n150 = local read "fMaxPlot"() -> (w493:dbl)
                n151 = local read "fMinPlot"() -> (w494:dbl)
                n152 = local read "fOversample"() -> (w488:dbl)
                n153 = local read "DecimFactor"() -> (w487:u32)
                n154 = local read "fSampleAcquire"() -> (w486:dbl)
                n155 = local read "Oversample"() -> (w489:bool)
                n156 = local read "Who"() -> (w496:string)
                n157 = local read "DeltaTAcquire"() -> (w485:dbl)
                n158 = local read "Pressure (t)"() -> (w483:sgl)
                n159 = local read "Name"() -> (w502:string)
                n160 = local read "Label"() -> (w503:string)
                n161 = Strip Path(path=w511) -> (stripped path=w517:path, name=w514:string)
                n162 = Number To Decimal String(number=w512, width (-)=2) -> (decimal integer string=w518:string)
                n163 = Format Date/Time String(time format string (%c)="%d %b %Y", seconds (now)=w508) -> (date/time string=w504:string)  [unwired: 1 out]
                n164 = Format Date/Time String(time format string (%c)="%H:%M:%S", seconds (now)=w508) -> (date/time string=w505:string)  [unwired: 1 out]
                n165 = call <vilib>:"Trim Whitespace.vi"("string"=w518) -> ("trimmed string"=w515:string)  [unwired: 1 in]
                n166 = Concatenate Strings(w514, "_", w515, ".txt") -> (w501:string)
                n167 = Build Path(base path=w517, name or relative path=w501) -> (appended path=w498:path)
                "DataFilePath" <- w498
                n168 = Format Into String(format string=w507, w501, w502, w503, w504, w505, w496, w506, w500, w495, w494, w493, w492, w490, w491, w489, w488, w487, w486, w485, w484, w483, "Comment") -> (resulting string=w499:string)  [unwired: 2 in, 1 out]
                "WriteNewHeader" <- FALSE
              }
              frame True {
                # "Exciter State"
                # "Date"
                # "Time"
                n169 = Format Date/Time String(time format string (%c)="%d %b %Y", seconds (now)=w522) -> (date/time string=w525:string)  [unwired: 1 out]
                n170 = Format Date/Time String(time format string (%c)="%H:%M:%S", seconds (now)=w522) -> (date/time string=w524:string)  [unwired: 1 out]
                n171 = local write "WriteNewHeader"(FALSE) -> ()
                n172 = Format Into String(format string="Date:\\t%s \\nTime:\\t %s \\n\\nTime (s)\\t  X (V) \\t Y (V) \\t     Sum (V) \\n-------- \\t---------\\t-------- \\t --------\\n\\n", w525, w524) -> (resulting string=w523:string)  [unwired: 2 in, 1 out]
              }
            }
            n173 = Negate(x=w145) -> (-x=w144:dbl)
            n174 = call-poly <vilib>:"DAQmx Create Virtual Channel.vi"("task in"=w143, "maximum value"=w145, "minimum value"=w144, "input terminal configuration"=w146, "physical channels"=w140, "units"=w141, "error in"=w142) -> ("task out"=w137:refnum<k21>, "error out"=w136:errorcluster)  [unwired: 7 in]
            n175 = local read "fSampleAcquire"() -> (w138:dbl)
            n176 = call-poly <vilib>:"DAQmx Timing.vi"("task/channels in"=w137, "sample mode"=w139, "rate"=w138, "error in"=w136) -> ("task out"=w134:refnum<k21>, "error out"=w135:errorcluster)  [unwired: 10 in]
            n177 = Merge Errors(w198, w135) -> (w133:errorcluster)
            n178 = local read "Excite"() -> (w197:bool)
            n179 = Unbundle By Name(w133) -> ("status"=w190:bool)
            n180 = case shown="True" w197 {
              tunnel: w200 -> [w530 w551]
              tunnel: w198 -> [w529 w550]
              tunnel: w166 -> [w533 w549]
              tunnel: w169 -> [w532 w548]
              tunnel: w168 -> [w531 w547]
              tunnel: w167 -> [w534 w545]
              frame False {
                n181 = Release Queue(queue=w534, error in (no error)=w533) -> ()  [unwired: 1 in, 3 out]
                n182 = Release Notifier(notifier=w532, error in (no error)=w531) -> ()  [unwired: 1 in, 3 out]
                n183 = call <vilib>:"DAQmx Clear Task.vi"("task in"=w530, "error in"=w529) -> ()  [unwired: 13 in, 1 out]
              }
              frame True {
                w546 = T8 4 items=["no dialog", "OK message", "continue or stop message", "OK message + warnings", "continue/stop + warnings"] ("type of dialog (OK msg:1)")
                # "Rezero Output"
                n184 = local read "nPlotPerRun"() -> (w557:u64)
                n185 = while {
                  tunnel: w548 -> [w606]
                  tunnel: w547 -> [w605]
                  i -> [w592]
                  stop <- w594 stop-if-true
                  # "Decimate Plot Data"
                  # "Plot Driving Waveform"
                  n186 = Wait on Notification(notifier=w606, error in (no error)=w605) -> (notification=w604:dbl[][], error out=w583:errorcluster)  [unwired: 2 in, 2 out]
                  n187 = local read "PlotPoints"() -> (w602:u32)
                  n188 = Reshape Array(w604, 1, w602) -> (w601:dbl[][])
                  n189 = local read "DecimFactor"() -> (w589:u32)
                  n190 = Index Array(array=w601, index (row)=0) -> (element=w587:dbl[])  [unwired: 1 in]
                  n191 = call-poly <vilib>:"Decimate (continuous).vi"("error in (no error)"=w583, "averaging"=TRUE, "decimating factor"=w589, "X"=w587) -> ("error out"=w584:errorcluster, "Decimated Array"=w586:dbl[])  [unwired: 6 in]
                  n192 = local read "DeltaTOutput"() -> (w599:dbl)
                  n193 = local read "Averaging"() -> (w585:T1)
                  n194 = Get Date/Time In Seconds() -> (seconds since 1Jan1904=w598:timestamp)
                  n195 = Bundle By Name("t0"=w598, "dt"=w599, "Y"=w586) -> (w597:waveform(dbl))  [unwired: 1 in]
                  n196 = call-poly <vilib>:"FFT Power Spectrum and PSD.vi"("averaging parameters"=w585, "error in (no error)"=w584, "time signal"=w597) -> ("error out"=w596:errorcluster, "Power Spectrum / PSD"=w576:cluster{"f0":dbl, "df":dbl, "magnitude":dbl[]})  [unwired: 5 in, 2 out]
                  n197 = Unbundle By Name(w596) -> ("status"=w595:bool)
                  n198 = local read "stop"() -> (w593:bool)
                  n199 = Unbundle(w576) -> ("f0"=w581:dbl, "df"=w578:dbl, "magnitude"=w577:dbl[])
                  n200 = Or(x=w595, y=w593) -> (x .or. y?=w594:bool)
                  n201 = Multiply(x=0.0, y=w577) -> (x*y=w579:dbl[])
                  n202 = local read "nPlotPerRun"() -> (w591:u64)
                  n203 = Build Array(w577, w579) -> (w580:dbl[][])
                  n204 = Bundle("f0"=w581, "df"=w578, w580) -> (w575:cluster{"f0":dbl, "df":dbl, dbl[][]})  [unwired: 1 in]
                  n205 = Less?(x=w592, y=w591) -> (x < y?=w590:bool)
                  n206 = case shown="True" w590 {
                    tunnel: w575 -> [_ w607]
                    frame False {
                    }
                    frame True {
                      n207 = local write "PSD Y"(w607) -> ()
                    }
                  }
                }
                n208 = while {
                  tunnel: w545 -> [w658]
                  tunnel: w549 -> [w654]
                  stop <- w650 stop-if-true
                  # "Driving Array"
                  # "Generate Driving Array"
                  n209 = local read "fSampleAcquire"() -> (w665:dbl)
                  n210 = local read "PlotPoints"() -> (w664:u32)
                  n211 = local read "High Pass IIR filter specs"() -> (w660:T2)
                  n212 = Bundle("fSampleAcquire"=w665, "PlotPoints"=w664) -> (w666:cluster{"fSampleAcquire":dbl, "PlotPoints":u32})  [unwired: 1 in]
                  n213 = call <vilib>:"Uniform White Noise Waveform.vi"("sampling info"=w666) -> ("error out"=w676:errorcluster, "signal out"=w675:waveform(dbl))  [unwired: 9 in]
                  n214 = call-poly <vilib>:"Digital IIR Filter.vi"("IIR filter specifications"=w660, "error in (no error)"=w676, "signal in"=w675) -> ("error out"=w674:errorcluster, "signal out"=w673:waveform(dbl))  [unwired: 6 in, 1 out]
                  n215 = call <vilib>:"Normalize Waveform.vi"("error in (no error)"=w674, "waveform in"=w673) -> ("error out"=w672:errorcluster, "normalized waveform"=w671:waveform(dbl))  [unwired: 6 in, 2 out]
                  n216 = call <vilib>:"Waveform Scale and Offset.vi"("error in (no error)"=w672, "scale"="Ampl. (V)", "offset"="Offset (V)", "waveform in"=w671) -> ("error out"=w653:errorcluster, "waveform out"=w667:waveform(dbl))  [unwired: 6 in]
                  n217 = local read "nBufferPerPlot"() -> (w663:u32)
                  n218 = local read "BufferPoints"() -> (w662:u32)
                  n219 = Unbundle By Name(w667) -> ("Y"=w668:dbl[])
                  n220 = Merge Errors(w654, w653) -> (w655:errorcluster)
                  n221 = Build Array(w668) -> (w677:dbl[][])
                  n222 = Reshape Array(w677, w663, w662) -> (w661:dbl[][])
                  n223 = local read "PlotPeriod"() -> (w656:dbl)
                  n224 = Enqueue Element(queue=w658, element=w661, error in (no error)=w655) -> (error out=w652:errorcluster)  [unwired: 1 in, 2 out]
                  n225 = Multiply(x=100.0, y=w656) -> (x*y=w659:dbl)
                  n226 = Unbundle By Name(w652) -> ("status"=w651:bool)
                  n227 = local read "stop"() -> (w649:bool)
                  n228 = Wait (ms)(milliseconds to wait=w659) -> ()  [unwired: 1 out]
                  n229 = Or(x=w651, y=w649) -> (x .or. y?=w650:bool)
                }
                n230 = while {
                  tunnel: w545 -> [w684]
                  tunnel: w549 -> [w683]
                  tunnel: [w679] -> w540
                  tunnel: [w678] -> w542
                  stop <- w681 stop-if-true
                  # "Drive Queue Element Check"
                  n231 = Get Queue Status(queue=w684, error in (no error)=w683) -> (queue out=w678:refnum<queue>, error out=w679:errorcluster, # elements in queue=→"# Elements Drive Queue":i32)  [unwired: 1 in, 5 out]
                  n232 = Unbundle By Name(w679) -> ("status"=w682:bool)
                  n233 = local read "stop"() -> (w680:bool)
                  n234 = Or(x=w682, y=w680) -> (x .or. y?=w681:bool)
                  n235 = Wait (ms)(milliseconds to wait=100) -> ()  [unwired: 1 out]
                }
                n236 = for {
                  N: w557 -> [_]
                  tunnel: w545 -> [w629]
                  tunnel: w549 -> [w628]
                  tunnel: w551 -> [w631]
                  tunnel: [w633] -> w555
                  tunnel: w550 -> [w630]
                  tunnel: [w632] -> w556
                  tunnel: w548 -> [w624]
                  tunnel: w547 -> [w623]
                  tunnel: [w622] -> w537
                  tunnel: [w621] -> w535
                  i -> [w618]
                  stop <- w625 stop-if-true
                  # "Zero the first write segment and record PSD.  Then subtract his PSD. background from  new data PSDs."
                  # "Write Output to Drive Exciter"
                  n237 = Dequeue Element(queue=w629, error in (no error)=w628) -> (element=w616:dbl[][], error out=w627:errorcluster)  [unwired: 1 in, 2 out]
                  n238 = Equal To 0?(x=w618) -> (x = 0?=w617:bool)
                  n239 = case shown="True" w617 {
                    tunnel: w616 -> [w634 w637]
                    tunnel: [w634 w635] -> w615
                    frame False {
                    }
                    frame True {
                      n240 = Multiply(x=0.0, y=w637) -> (x*y=w635:dbl[][])
                    }
                  }
                  n241 = for {
                    tunnel: w631 -> [w638]
                    tunnel: w630 -> [w641]
                    tunnel: [w643] -> w633
                    tunnel: [w642] -> w632
                    tunnel: w615 -> [w645] mode=indexing
                    stop <- w647 stop-if-true
                    n242 = Build Array(w645) -> (w639:dbl[][])
                    n243 = local read "BufferPeriod"() -> (w646:dbl)
                    n244 = call-poly <vilib>:"DAQmx Write.vi"("task/channels in"=w638, "data"=w639, "timeout"=10.0, "error in"=w641) -> ("task out"=w643:refnum<k21>, "error out"=w642:errorcluster)  [unwired: 9 in, 1 out]
                    n245 = Unbundle By Name(w642) -> ("status"=w648:bool)
                    n246 = local read "stop"() -> (w644:bool)
                    n247 = Wait (ms)(milliseconds to wait=w646) -> ()  [unwired: 1 out]
                    n248 = Or(x=w648, y=w644) -> (x .or. y?=w647:bool)
                  }
                  n249 = Send Notification(notification=w615, notifier=w624, error in (no error)=w623) -> (notifier out=w621:refnum<notifier>, error out=w622:errorcluster)
                  n250 = Merge Errors(w632, w627, w622) -> (w626:errorcluster)
                  n251 = Unbundle By Name(w626) -> ("status"=w620:bool)
                  n252 = local read "stop"() -> (w619:bool)
                  n253 = Or(x=w619, y=w620) -> (x .or. y?=w625:bool)
                }
                n254 = local read "ReZero"() -> (w554:dbl[][])
                n255 = for {
                  tunnel: w554 -> [w613] mode=indexing
                  tunnel: w556 -> [w612]
                  tunnel: w555 -> [w610]
                  tunnel: [w609] -> w553
                  tunnel: [w608] -> w552
                  n256 = local read "BufferPeriod"() -> (w614:dbl)
                  n257 = Build Array(w613) -> (w611:dbl[][])
                  n258 = call-poly <vilib>:"DAQmx Write.vi"("task/channels in"=w610, "data"=w611, "error in"=w612) -> ("task out"=w609:refnum<k21>, "error out"=w608:errorcluster)  [unwired: 10 in, 1 out]
                  n259 = Wait (ms)(milliseconds to wait=w614) -> ()  [unwired: 1 out]
                }
                n260 = flat-sequence {
                  tunnel: w553 -> [w562]
                  tunnel: w552 -> [w561]
                  tunnel: [w558] -> w543
                  tunnel: w542 -> [w566]
                  tunnel: [w566] -> w541
                  tunnel: w540 -> [w565]
                  tunnel: [w565] -> w539
                  tunnel: [w564] -> w538
                  tunnel: w537 -> [w564]
                  tunnel: [w563] -> w536
                  tunnel: w535 -> [w563]
                  tunnel: [w570] -> w544
                  tunnel: w543 -> [w568]
                  tunnel: w541 -> [w574]
                  tunnel: w539 -> [w573]
                  tunnel: w538 -> [w572]
                  tunnel: w536 -> [w571]
                  frame #0 {
                    n261 = call <vilib>:"DAQmx Stop Task.vi"("task/channels in"=w562, "error in"=w561) -> ("task out"=w560:refnum<k21>, "error out"=w559:errorcluster)  [unwired: 12 in]
                    n262 = call <vilib>:"DAQmx Clear Task.vi"("task in"=w560, "error in"=w559) -> ("error out"=w558:errorcluster)  [unwired: 13 in]
                  }
                  frame #1 {
                    n263 = Release Queue(queue=w574, error in (no error)=w573) -> (error out=w567:errorcluster)  [unwired: 1 in, 2 out]
                    n264 = Release Notifier(notifier=w571, error in (no error)=w572) -> (error out=w569:errorcluster)  [unwired: 1 in, 2 out]
                    n265 = Merge Errors(w567, w568, w569) -> (w570:errorcluster)
                  }
                }
                n266 = call <vilib>:"Simple Error Handler.vi"("type of dialog (OK msg:1)"=w546, "error in (no error)"=w544) -> ()  [unwired: 3 in, 5 out]
              }
            }
            n267 = local write "stop"(w190) -> ()
            n268 = Open/Create/Replace File(file path (use dialog)=w195, operation (0:open)=T5."create", access (0:read/write)=enum16{"read/write", "read-only", "write-only"}."write-only") -> (refnum out=w158:refnum<file>, error out=w208:errorcluster)  [unwired: 1 in, 3 out]
            n269 = call <vilib>:"DAQmx Start Task.vi"("task/channels in"=w134, "error in"=w133) -> ("task out"=w131:refnum<k21>, "error out"=w132:errorcluster)  [unwired: 12 in]
            n270 = Refnum to Path(1:w158) -> (0:→"PathAtOpen":path)
            n271 = Write to Text File(file (use dialog)=w158, text=w205, error in=w208) -> (refnum out=w181:refnum<file>)  [unwired: 3 out]
            n272 = local read "nPlotPerRun"() -> (w203:u64)
            n273 = while {
              tunnel: w155 -> [w366]
              tunnel: w154 -> [w365]
              i -> [w333]
              stop <- w367 stop-if-true
              w347 = -0.9033  # CY1
              w348 = 0.1954  # CY2
              w349 = 0.2371  # CX2
              w350 = -0.8847  # CX1
              # "Y"
              # "X"
              # "Plot Data"
              n274 = Wait on Notification(notifier=w366, error in (no error)=w365) -> (notification=w370:dbl[][], error out=w369:errorcluster)  [unwired: 2 in, 2 out]
              n275 = Transpose 2D Array(2D array=w370) -> (transposed array=w381:dbl[][])
              n276 = Index Array(array=w381, index (row) #1=1, index (row) #2=2, index (row) #3=3) -> (element #1=w376:dbl[], element #2=w374:dbl[], element #3=w375:dbl[])  [unwired: 3 in]
              n277 = Divide(x=w376, y=w375) -> (x/y=w352:dbl[])
              n278 = Divide(x=w374, y=w375) -> (x/y=w353:dbl[])
              n279 = property on="Unit" class="Ring (strict)"() -> ("Value"=w345:u16)  [unwired: 2 in, 2 out]
              n280 = Multiply(x="LeverArm (m)", y=1000.0) -> (x*y=w340:dbl)
              n281 = case shown="0, Default" w345 {
                selector: w345 -> [w402 w405 w431 w457]
                tunnel: w353 -> [w403 w428 w455 w472]
                tunnel: w352 -> [w404 w414 w453 w470]
                tunnel: [w403 w420 w454 w471] -> w351
                tunnel: [w404 w411 w429 w462] -> w338
                tunnel: w350 -> [_ w410 w452 w469]
                tunnel: w349 -> [_ w409 w451 w468]
                tunnel: w348 -> [_ w408 w430 w467]
                tunnel: w340 -> [_ w407 w450 w466]
                tunnel: w347 -> [_ w406 w449 w465]
                frame 0, Default {
                  n282 = local write "PlotUnitIndex"(w402) -> ()
                }
                frame 1 {
                  n283 = Divide(x=w414, y=w410) -> (x/y=w419:dbl[])
                  n284 = Divide(x=w409, y=w407) -> (x/y=w412:dbl)
                  n285 = Divide(x=w408, y=w407) -> (x/y=w421:dbl)
                  n286 = Divide(x=w428, y=w406) -> (x/y=w427:dbl[])
                  n287 = local write "PlotUnitIndex"(w405) -> ()
                  n288 = Increment(x=w419) -> (x+1=w416:dbl[])
                  n289 = Decrement(x=w419) -> (x-1=w418:dbl[])
                  n290 = Increment(x=w427) -> (x+1=w424:dbl[])
                  n291 = Decrement(x=w427) -> (x-1=w426:dbl[])
                  n292 = Negate(x=w418) -> (-x=w417:dbl[])
                  n293 = Negate(x=w426) -> (-x=w425:dbl[])
                  n294 = Divide(x=w424, y=w425) -> (x/y=w423:dbl[])
                  n295 = Divide(x=w416, y=w417) -> (x/y=w415:dbl[])
                  n296 = Natural Logarithm(1:w423) -> (0:w422:dbl[])
                  n297 = Natural Logarithm(1:w415) -> (0:w413:dbl[])
                  n298 = Multiply(x=w413, y=w412) -> (x*y=w411:dbl[])
                  n299 = Multiply(x=w421, y=w422) -> (x*y=w420:dbl[])
                }
                frame 2 {
                  w439 = 2.0
                  n300 = Divide(x=w455, y=w449) -> (x/y=w434:dbl[])
                  n301 = Divide(x=w453, y=w452) -> (x/y=w444:dbl[])
                  n302 = Square(x=w434) -> (x^2=w438:dbl[])
                  n303 = Divide(x=w451, y=w450) -> (x/y=w443:dbl)
                  n304 = Divide(x=w430, y=w450) -> (x/y=w440:dbl)
                  n305 = Square(x=w444) -> (x^2=w448:dbl[])
                  n306 = Divide(x=w438, y=3.0) -> (x/y=w436:dbl[])
                  n307 = Divide(x=w448, y=3.0) -> (x/y=w446:dbl[])
                  n308 = Multiply(x=w443, y=w439) -> (x*y=w442:dbl)
                  n309 = Multiply(x=w439, y=w440) -> (x*y=w432:dbl)
                  n310 = Increment(x=w436) -> (x+1=w435:dbl[])
                  n311 = Increment(x=w446) -> (x+1=w445:dbl[])
                  n312 = Multiply(x=w435, y=w434) -> (x*y=w433:dbl[])
                  n313 = Multiply(x=w445, y=w444) -> (x*y=w441:dbl[])
                  n314 = Multiply(x=w432, y=w433) -> (x*y=w454:dbl[])
                  n315 = Multiply(x=w441, y=w442) -> (x*y=w429:dbl[])
                  "PlotUnitIndex" <- w431
                }
                frame 3 {
                  w460 = 2.0
                  n316 = local write "PlotUnitIndex"(w457) -> ()
                  n317 = Divide(x=w470, y=w469) -> (x/y=w458:dbl[])
                  n318 = Divide(x=w472, y=w465) -> (x/y=w456:dbl[])
                  n319 = Divide(x=w468, y=w466) -> (x/y=w464:dbl)
                  n320 = Divide(x=w467, y=w466) -> (x/y=w461:dbl)
                  n321 = Multiply(x=w464, y=w460) -> (x*y=w463:dbl)
                  n322 = Multiply(x=w460, y=w461) -> (x*y=w459:dbl)
                  n323 = Multiply(x=w458, y=w463) -> (x*y=w462:dbl[])
                  n324 = Multiply(x=w459, y=w456) -> (x*y=w471:dbl[])
                }
              }
              n325 = local read "DeltaTOutput"() -> (w379:dbl)
              n326 = Array Size(array=w338) -> (size(s)=→"SizeTimeSeries":i32)
              n327 = Get Date/Time In Seconds() -> (seconds since 1Jan1904=w380:timestamp)
              n328 = Bundle By Name("t0"=w380, "dt"=w379, "Y"=w351) -> (w378:waveform(dbl))  [unwired: 1 out]
              n329 = Bundle By Name("t0"=w380, "dt"=w379, "Y"=w338) -> (w377:waveform(dbl))  [unwired: 1 out]
              n330 = property on="Type" class="Ring (strict)"() -> ("Value"=w346:u16)  [unwired: 2 in, 2 out]
              n331 = call-poly <vilib>:"FFT Power Spectrum and PSD.vi"("export mode"=w346, "averaging parameters"="Averaging", "time signal"=w378) -> ("error out"=w382:errorcluster, "Power Spectrum / PSD"=w362:cluster{"f0":dbl, "df":dbl, "magnitude":dbl[]})  [unwired: 5 in, 2 out]
              n332 = call-poly <vilib>:"FFT Power Spectrum and PSD.vi"("export mode"=w346, "averaging parameters"="Averaging", "time signal"=w377) -> ("error out"=w383:errorcluster, "averages completed"=→"NAve":dbl, "Power Spectrum / PSD"=w363:cluster{"f0":dbl, "df":dbl, "magnitude":dbl[]})  [unwired: 5 in, 1 out]
              n333 = Merge Errors(w383, w382, w369) -> (w368:errorcluster)
              n334 = Unbundle By Name(w363) -> ("f0"=w357:dbl, "df"=w339:dbl, "magnitude"=w344:dbl[])
              "df" <- w339
              n335 = Unbundle By Name(w362) -> ("magnitude"=w343:dbl[])  [unwired: 2 out]
              n336 = Unbundle By Name(w368) -> ("status"=w360:bool)
              n337 = local read "stop"() -> (w359:bool)
              n338 = Square Root(x=w344) -> (sqrt(x)=w330:dbl[])
              n339 = Square Root(x=w343) -> (sqrt(x)=w331:dbl[])
              n340 = Or(x=w359, y=w360) -> (x .or. y?=w367:bool)
              n341 = Equal To 0?(x=w333) -> (x = 0?=w332:bool)
              n342 = case shown="True" w332 {
                tunnel: w331 -> [_ w401]
                tunnel: w330 -> [_ w392]
                frame False {
                }
                frame True {
                  n343 = Array Max & Min(array=w401) -> (max value=w398:dbl, min value=w393:dbl)  [unwired: 2 out]
                  n344 = Array Max & Min(array=w392) -> (max value=w391:dbl, min value=w386:dbl)  [unwired: 2 out]
                  n345 = Logarithm Base 10(1:w398) -> (0:w397:dbl)
                  n346 = Logarithm Base 10(1:w391) -> (0:w390:dbl)
                  n347 = Round Toward +Infinity(x=w397) -> (ceil(x): smallest int >= x=w396:dbl)
                  n348 = Round Toward +Infinity(x=w390) -> (ceil(x): smallest int >= x=w389:dbl)
                  n349 = Power Of 10(x=w396) -> (10^x=w394:dbl)
                  n350 = Power Of 10(x=w389) -> (10^x=w384:dbl)
                  n351 = property on="PSD Y" class="WFGraph (strict)"("YScale.Maximum"=w394) -> ()  [unwired: 2 in, 2 out]
                  n352 = property on="PSD X" class="WFGraph (strict)"("YScale.Maximum"=w384) -> ()  [unwired: 2 in, 2 out]
                  n353 = Logarithm Base 10(1:w393) -> (0:w400:dbl)
                  n354 = Logarithm Base 10(1:w386) -> (0:w388:dbl)
                  n355 = Round Toward -Infinity(1:w400) -> (0:w399:dbl)
                  n356 = Round Toward -Infinity(1:w388) -> (0:w387:dbl)
                  n357 = Power Of 10(x=w399) -> (10^x=w395:dbl)
                  n358 = Power Of 10(x=w387) -> (10^x=w385:dbl)
                  n359 = property on="PSD Y" class="WFGraph (strict)"("YScale.Minimum"=w395) -> ()  [unwired: 2 in, 2 out]
                  n360 = property on="PSD X" class="WFGraph (strict)"("YScale.Minimum"=w385) -> ()  [unwired: 2 in, 2 out]
                }
              }
              n361 = Build Array(w330, w331) -> (w335:dbl[][])
              n362 = Build Array(w331, w330) -> (w334:dbl[][])
              n363 = Bundle("f0"=w357, "df"=w339, w334) -> (w354:cluster{"f0":dbl, "df":dbl, dbl[][]})  [unwired: 1 in]
              n364 = Bundle("f0"=w357, "df"=w339, w335) -> (w355:cluster{"f0":dbl, "df":dbl, dbl[][]})  [unwired: 1 in]
              n365 = Bundle("f0"=w357, "df"=w339, w335) -> (w356:cluster{"f0":dbl, "df":dbl, dbl[][]})  [unwired: 1 in]
              n366 = local read "nPlotPerRun"() -> (w358:u64)
              n367 = Less?(x=w333, y=w358) -> (x < y?=w364:bool)
              n368 = case shown="True" w364 {
                tunnel: w356 -> [_ w473]
                tunnel: w355 -> [_ w475]
                tunnel: w354 -> [_ w474]
                frame False {
                }
                frame True {
                  n369 = local write "Plot1"(w473) -> ()
                  n370 = local write "Plot2"(w473) -> ()
                  n371 = local write "Plot3"(w473) -> ()
                  n372 = local write "Plot4"(w473) -> ()
                  n373 = local read "Excite"() -> (w476:bool)
                  n374 = local write "Plot5"(w473) -> ()
                  n375 = local write "Plot6"(w473) -> ()
                  n376 = local write "Plot7"(w473) -> ()
                  n377 = local write "Plot8"(w473) -> ()
                  n378 = case shown="False" w476 {
                    tunnel: w475 -> [w477 w479]
                    tunnel: w474 -> [w478 _]
                    frame False {
                      n379 = local write "PSD Y"(w478) -> ()
                      n380 = property on="PSD X" class="WFGraph (strict)"("Val(Sgnl)"=w477) -> ()  [unwired: 2 in, 2 out]
                    }
                    frame True {
                      n381 = local write "PSD X"(w479) -> ()
                    }
                  }
                }
              }
              "Plot" <- w333
            }
            n382 = while {
              tunnel: w181 -> [w245]
              tunnel: w155 -> [w242]
              tunnel: w154 -> [w241]
              tunnel: w157 -> [w240]
              tunnel: w156 -> [w239]
              i -> [w223]
              stop <- w243 stop-if-true
              # "DATA\nTime\nX\nY\nSUM"
              # "Write to Temp/Data File"
              n383 = Dequeue Element(queue=w240, error in (no error)=w239) -> (element=w227:dbl[][], error out=w229:errorcluster)  [unwired: 1 in, 2 out]
              n384 = local read "Input Data Type"() -> (w230:u16)
              n385 = Array Size(array=w227) -> (size(s)=→"Raw Data Size":i32[])
              n386 = case shown="2" w230 {
                tunnel: w229 -> [w249 w274 w294]
                tunnel: w227 -> [w248 w277 w297]
                tunnel: [w249 w274 w294] -> w228
                tunnel: [w248 w272 w292] -> w224
                frame 0, Default {
                }
                frame 1 {
                  # "Time\nQ 1+/-  —  4+/-"
                  # "Time\nX\nY\nSUM"
                  n387 = Index Array(array=w277, index (col) #1=0, index (col) #2=1, index (col) #3=2, index (col) #4=3, index (col) #5=4, index (col) #6=5, index (col) #7=6, index (col) #8=7, index (col) #9=8) -> (element #1=w275:dbl[], element #2=w261:dbl[], element #3=w260:dbl[], element #4=w259:dbl[], element #5=w258:dbl[], element #6=w257:dbl[], element #7=w256:dbl[], element #8=w263:dbl[], element #9=w262:dbl[])  [unwired: 9 in]
                  n388 = Subtract(x=w261, y=w260) -> (x-y=w254:dbl[])
                  n389 = Subtract(x=w259, y=w258) -> (x-y=w253:dbl[])
                  n390 = Subtract(x=w257, y=w256) -> (x-y=w255:dbl[])
                  n391 = Subtract(x=w263, y=w262) -> (x-y=w252:dbl[])
                  n392 = Subtract(x=w254, y=w253) -> (x-y=w250:dbl[])
                  n393 = Subtract(x=w255, y=w252) -> (x-y=w251:dbl[])
                  n394 = Compound Arithmetic op=ADD(w254, w253, w255, w252) -> (w268:dbl[])
                  n395 = Add(x=w250, y=w251) -> (x+y=w271:dbl[])
                  n396 = Subtract(x=w250, y=w251) -> (x-y=w270:dbl[])
                  n397 = Negate(x=w271) -> (-x=w269:dbl[])
                  n398 = Build Array(w275, w270, w269, w268) -> (w273:dbl[][])
                  n399 = Transpose 2D Array(2D array=w273) -> (transposed array=w272:dbl[][])
                }
                frame 2 {
                  # "Time\nQ 1 —  4"
                  # "Time\nX\nY\nSUM"
                  n400 = Index Array(array=w297, index (col) #1=0, index (col) #2=1, index (col) #3=2, index (col) #4=3, index (col) #5=4) -> (element #1=w295:dbl[], element #2=w285:dbl[], element #3=w284:dbl[], element #4=w283:dbl[], element #5=w282:dbl[])  [unwired: 5 in]
                  n401 = Subtract(x=w285, y=w284) -> (x-y=w286:dbl[])
                  n402 = Subtract(x=w283, y=w282) -> (x-y=w287:dbl[])
                  n403 = Compound Arithmetic op=ADD(w285, w284, w283, w282) -> (w288:dbl[])
                  n404 = Add(x=w286, y=w287) -> (x+y=w291:dbl[])
                  n405 = Subtract(x=w286, y=w287) -> (x-y=w290:dbl[])
                  n406 = Negate(x=w291) -> (-x=w289:dbl[])
                  n407 = Build Array(w295, w290, w289, w288) -> (w293:dbl[][])
                  n408 = Transpose 2D Array(2D array=w293) -> (transposed array=w292:dbl[][])
                }
              }
              n409 = Array Size(array=w224) -> (size(s)=→"Converted Data Size":i32[])
              n410 = local read "Oversample"() -> (w231:bool)
              n411 = Equal To 0?(x=w223) -> (x = 0?=w222:bool)
              n412 = case shown="True" w231 {
                tunnel: w224 -> [w303 w311]
                tunnel: [w303 w309] -> w235
                tunnel: [w302 w306] -> w233
                tunnel: w228 -> [w302 w307]
                tunnel: w222 -> [_ w304]
                frame False {
                }
                frame True {
                  w319 = TRUE
                  n413 = local read "DecimFactor"() -> (w320:u32)
                  n414 = Index Array(array=w311, index (col) #1=0, index (col) #2=1, index (col) #3=2, index (col) #4=3) -> (element #1=w323:dbl[], element #2=w305:dbl[], element #3=w322:dbl[], element #4=w321:dbl[])  [unwired: 4 in]
                  n415 = call-poly <vilib>:"Decimate (continuous).vi"("reset"=w304, "averaging"=w319, "decimating factor"=w320, "X"=w305) -> ("error out"=w314:errorcluster, "Decimated Array"=w308:dbl[])  [unwired: 6 in]
                  n416 = call-poly <vilib>:"Decimate (continuous).vi"("reset"=w304, "averaging"=w319, "decimating factor"=w320, "X"=w322) -> ("error out"=w312:errorcluster, "Decimated Array"=w317:dbl[])  [unwired: 6 in]
                  n417 = call-poly <vilib>:"Decimate (continuous).vi"("reset"=w304, "averaging"=w319, "decimating factor"=w320, "X"=w321) -> ("error out"=w315:errorcluster, "Decimated Array"=w316:dbl[])  [unwired: 6 in]
                  n418 = call-poly <vilib>:"Decimate (continuous).vi"("reset"=w304, "averaging"=w319, "decimating factor"=w320, "X"=w323) -> ("error out"=w313:errorcluster, "Decimated Array"=w318:dbl[])  [unwired: 6 in]
                  n419 = Build Array(w318, w308, w317, w316) -> (w310:dbl[][])
                  n420 = Merge Errors(w313, w314, w312, w315, w307) -> (w306:errorcluster)
                  n421 = Transpose 2D Array(2D array=w310) -> (transposed array=w309:dbl[][])
                }
              }
              n422 = local read "nPlotPerRun"() -> (w237:u64)
              "WriteLimit" <- w237
              n423 = Send Notification(notification=w235, notifier=w242, error in (no error)=w241) -> (error out=w232:errorcluster)  [unwired: 1 out]
              n424 = Array To Spreadsheet String(array=w235, 3:"%.6f") -> (spreadsheet string=w246:string)  [unwired: 1 in]
              n425 = Merge Errors(w233, w232) -> (w234:errorcluster)
              n426 = Less?(x=w223, y=w237) -> (x < y?=w236:bool)
              n427 = case shown="True" w236 {
                tunnel: w246 -> [_ w329]
                tunnel: w245 -> [_ w328]
                frame False {
                }
                frame True {
                  n428 = Write to Text File(file (use dialog)=w328, text=w329) -> ()  [unwired: 2 in, 3 out]
                }
              }
              n429 = Unbundle By Name(w234) -> ("status"=w244:bool)
              n430 = local read "stop"() -> (w238:bool)
              n431 = Or(x=w244, y=w238) -> (x .or. y?=w243:bool)
              "WriteNumber" <- w223
            }
            n432 = while {
              tunnel: w157 -> [w858]
              tunnel: w156 -> [w857]
              stop <- w854 stop-if-true
              # "Response Queue Element Check"
              n433 = Get Queue Status(queue=w858, error in (no error)=w857) -> (error out=w853:errorcluster, # elements in queue=→"# Elements Response Queue":i32)  [unwired: 1 in, 6 out]
              n434 = Unbundle By Name(w853) -> ("status"=w856:bool)
              n435 = local read "stop"() -> (w855:bool)
              n436 = Or(x=w855, y=w856) -> (x .or. y?=w854:bool)
              n437 = Wait (ms)(milliseconds to wait=100) -> ()  [unwired: 1 out]
            }
            n438 = for {
              N: w203 -> [_]
              tunnel: w131 -> [w826]
              tunnel: [w827] -> w193
              tunnel: w132 -> [w825]
              tunnel: [w819] -> w192
              tunnel: w157 -> [w813]
              tunnel: w156 -> [w812]
              i -> [w817]
              stop <- w815 stop-if-true
              # "Read Sample Data"
              n439 = local read "PlotPeriod"() -> (w818:dbl)
              n440 = local read "nBufferPerPlot"() -> (w822:u32)
              n441 = Multiply(x=w817, y=w818) -> (x*y=w816:dbl)
              n442 = for {
                N: w822 -> [_]
                shift-right: [w832] -> w827
                shift-left: w826 -> [w833]
                shift-right: [w831] -> w819
                shift-left: w825 -> [w834]
                tunnel: [w845] -> w821 mode=concatenating
                tunnel: w816 -> [w840]
                i -> [w843]
                stop <- w846 stop-if-true
                n443 = local read "BufferPeriod"() -> (w844:dbl)
                n444 = local read "BufferPoints"() -> (w829:u32)
                n445 = local read "time vector"() -> (w839:dbl[])
                n446 = Multiply(x=w843, y=w844) -> (x*y=w842:dbl)
                n447 = call-poly <vilib>:"DAQmx Read.vi"("task/channels in"=w833, "number of samples per channel"=w829, "timeout"=10.0, "error in"=w834) -> ("task out"=w832:refnum<k21>, "data"=w830:dbl[][], "error out"=w831:errorcluster)  [unwired: 9 in]
                n448 = Add(x=w842, y=w840) -> (x+y=w836:dbl)
                n449 = Add(x=w836, y=w839) -> (x+y=w838:dbl[])
                n450 = Greater Than 0?(x=w836) -> (x > 0?=w837:bool)
                n451 = Unbundle By Name(w831) -> ("status"=w847:bool)
                n452 = case shown="True" w837 {
                  tunnel: w836 -> [_ w852]
                  frame False {
                  }
                  frame True {
                    n453 = local read "RunPeriod"() -> (w849:dbl)
                    n454 = Multiply(x=w852, y=100) -> (x*y=w848:dbl)
                    n455 = Divide(x=w848, y=w849) -> (x/y=→"Progress":dbl)
                  }
                }
                n456 = Build Array (concatenate)(w838, w830) -> (w841:dbl[][])
                n457 = local read "stop"() -> (w835:bool)
                n458 = Transpose 2D Array(2D array=w841) -> (transposed array=w845:dbl[][])
                n459 = Or(x=w847, y=w835) -> (x .or. y?=w846:bool)
              }
              n460 = Enqueue Element(queue=w813, element=w821, error in (no error)=w812) -> (error out=w820:errorcluster)  [unwired: 1 in, 2 out]
              n461 = Merge Errors(w819, w820) -> (w824:errorcluster)
              n462 = Unbundle By Name(w824) -> ("status"=w823:bool)
              n463 = local read "stop"() -> (w814:bool)
              n464 = Or(x=w823, y=w814) -> (x .or. y?=w815:bool)
            }
            n465 = flat-sequence {
              tunnel: [w724] -> w194
              tunnel: w193 -> [w728]
              tunnel: w192 -> [w727]
              tunnel: w158 -> [w729]
              tunnel: [w729] -> w178
              tunnel: w194 -> [w736]
              tunnel: [w736] -> w191
              tunnel: [w735] -> w179
              tunnel: w178 -> [w735]
              tunnel: w191 -> [w742]
              tunnel: [w742] -> w183
              tunnel: [w741] -> w180
              tunnel: w179 -> [w741]
              tunnel: w183 -> [w743]
              tunnel: w180 -> [w760]
              tunnel: [w759] -> w153
              tunnel: w153 -> [w766]
              tunnel: [w762] -> w150
              tunnel: [w761] -> w151
              frame #0 {
                n466 = Refnum to Path(1:w729) -> (0:→"PathAtClose":path)
                n467 = call <vilib>:"DAQmx Stop Task.vi"("task/channels in"=w728, "error in"=w727) -> ("task out"=w726:refnum<k21>, "error out"=w725:errorcluster)  [unwired: 12 in]
                n468 = Wait (ms)(milliseconds to wait=1000) -> ()  [unwired: 1 out]
                n469 = call <vilib>:"DAQmx Clear Task.vi"("task in"=w726, "error in"=w725) -> ("error out"=w724:errorcluster)  [unwired: 13 in]
                "Step" <- 1
              }
              frame #1 {
                n470 = local write "Step"(2) -> ()
                n471 = local write "stop"(TRUE) -> ()
              }
              frame #2 {
                n472 = local read "PlotPeriod"() -> (w738:dbl)
                n473 = local write "Step"(3) -> ()
                n474 = Multiply(x=w738, y=1000) -> (x*y=w737:dbl)
                n475 = Wait (ms)(milliseconds to wait=w737) -> ()  [unwired: 1 out]
              }
              frame #3 {
                w746 = TRUE
                n476 = local write "Step"(4) -> ()
                n477 = Initialize Array(0.0, 1, 3) -> (w756:dbl[][])
                n478 = Close File(refnum=w760, error in=w743) -> (error out=w758:errorcluster)  [unwired: 1 out]
                n479 = Obtain Queue(name (unnamed)="Response Queue", element data type=w756) -> (queue out=w753:refnum<queue>, error out=w755:errorcluster)  [unwired: 3 in, 1 out]
                n480 = Obtain Notifier(name (unnamed)="Response Notifier", notification data type=w756) -> (notifier out=w752:refnum<notifier>, error out=w754:errorcluster)  [unwired: 2 in, 1 out]
                n481 = Release Queue(queue=w753, force destroy? (F)=w746, error in (no error)=w755) -> (error out=w745:errorcluster)  [unwired: 2 out]
                n482 = Release Notifier(notifier=w752, force destroy? (F)=w746, error in (no error)=w754) -> (error out=w744:errorcluster)  [unwired: 2 out]
                n483 = Merge Errors "Merge Errors"(w758, w745, w744) -> (w759:errorcluster)
              }
              frame #4 {
                w765 = T8 4 items=["no dialog", "OK message", "continue/stop", "OK + warnings", "cont./stop + warn"] ("type of dialog (OK msg:1)")
                n484 = local read "Excite"() -> (w768:bool)
                n485 = call <vilib>:"Simple Error Handler.vi"("type of dialog (OK msg:1)"=w765, "error in (no error)"=w766) -> ("error?"=w767:bool)  [unwired: 3 in, 4 out]
                n486 = local write "Step"(5) -> ()
                n487 = Or(x=w768, y=w767) -> (x .or. y?=w764:bool)
                n488 = case shown="False" w764 {
                  tunnel: [w771 2] -> w761
                  tunnel: [w770 FALSE] -> w762
                  frame False {
                    n489 = case shown="True" "AutoSave" {
                      tunnel: [0 w776] -> w771
                      tunnel: [FALSE w777] -> w770
                      frame False {
                        n490 = property on="Out" class="Path"("Val(Sgnl)"=path "") -> ()  [unwired: 2 in, 2 out]
                        n491 = property on="File" class="Str"("Val(Sgnl)"="") -> ()  [unwired: 2 in, 2 out]
                      }
                      frame True {
                        n492 = Format Into String(format string="\\n\\n%s\\n%s\\n%s", initial string="Check the parameters in the blue panel. ", "\"Save\" = Save immediately", "\"Change, then Save\" = Update Parameters, then press Save", "\"Cancel\" = Don't Save.") -> (resulting string=w779:string)  [unwired: 1 in, 1 out]
                        n493 = call <vilib>:"Three Button Dialog.vi"("Window Title (\"\")"="Parameter Check ", "Center Button Text (\"No\")"="Change, then Save", "Left Button Text (\"Yes\")"="Save", "message"=w779) -> ("Which Button?"=w778:T9)  [unwired: 2 in, 5 out]
                        n494 = case shown="\"Left Button\", Default" w778 {
                          tunnel: [FALSE FALSE FALSE FALSE] -> w777
                          tunnel: [2 0 2 2] -> w776
                          frame "Left Button", Default {
                            n495 = property on="Write Light" class="Bool (strict)"("Val(Sgnl)"=TRUE) -> ()  [unwired: 2 in, 2 out]
                            n496 = local write "WriteNewHeader"(FALSE) -> ()
                          }
                          frame "Center Button" {
                            n497 = property on="Out" class="Path"("Val(Sgnl)"=path "") -> ()  [unwired: 2 in, 2 out]
                            n498 = local write "WriteNewHeader"(TRUE) -> ()
                          }
                          frame "Right Button" {
                            # "\"Cancel\" = Don't Save."
                            n499 = local read "TempFilePath"() -> (w796:path)
                            n500 = local read "DataFilePath"() -> (w797:path)
                            n501 = property on="Out" class="Path"("Val(Sgnl)"=path "") -> ()  [unwired: 2 in, 2 out]
                            n502 = Move(source path=w797, 10:w796) -> ()  [unwired: 3 in, 3 out]
                          }
                          frame "Window Close" {
                            # "\"Cancel\" = Don't Save."
                            n503 = local read "TempFilePath"() -> (w802:path)
                            n504 = local read "DataFilePath"() -> (w801:path)
                            n505 = property on="Out" class="Path"("Val(Sgnl)"=path "") -> ()  [unwired: 2 in, 2 out]
                            n506 = Move(source path=w801, 10:w802) -> ()  [unwired: 3 in, 3 out]
                          }
                        }
                      }
                    }
                  }
                  frame True {
                    n507 = property on="Out" class="Path"("Val(Sgnl)"=path "") -> ()  [unwired: 2 in, 2 out]
                  }
                }
              }
            }
            n508 = Boolean To (0,1)(Boolean=w150) -> (0, 1=w152:i16)
            n509 = property on="Manual Save" class="Bool (strict)"("DisabledEnum"=w151) -> ()  [unwired: 2 in, 2 out]
            n510 = property on="RunLight" class="Bool (strict)"("Value"=w150) -> ()  [unwired: 2 in, 2 out]
            n511 = local write "stop"(w150) -> ()
            n512 = property on="Start" class="Bool (strict)"("Value"=w150) -> ()  [unwired: 2 in, 2 out]
            n513 = local write "Progress"(w152) -> ()
          }
          event "Offset (V)", "Ampl. (V)": Value Change {
            n514 = event-data() -> ()  [unwired: 7 out]
            n515 = local read "Ampl. (V)"() -> (w868:sgl)
            n516 = local read "Offset (V)"() -> (w867:sgl)
            n517 = Absolute Value(x=w867) -> (abs(x)=w864:sgl)
            n518 = Absolute Value(x=w868) -> (abs(x)=w862:sgl)
            n519 = Add(x=w864, y=w862) -> (x+y=w866:sgl)
            n520 = local read "Max Value"() -> (w863:dbl)
            n521 = Greater?(x=w866, y=w863) -> (0:w865:bool)
            n522 = Subtract(x=w863, y=w862) -> (x-y=w861:dbl)
            n523 = case shown="True" w865 {
              tunnel: w861 -> [_ w869]
              frame False {
              }
              frame True {
                n524 = local write "Offset (V)"(w869) -> ()
              }
            }
          }
          event "Averaging.weighting mode": Value Change {
            n525 = event-data() -> ()  [unwired: 7 out]
            n526 = property on="Averaging" class="Clust (strict)"() -> ("Value"=w875:T1)  [unwired: 2 in, 2 out]
            n527 = Unbundle By Name(w875) -> ("Averaging"=w874:T6, "weighting mode"=w870:enum16{"Linear", "Exponential"})  [unwired: 1 out]
            n528 = Equal To 0?(x=w870) -> (x = 0?=w872:bool)
            n529 = case shown="True" w872 {
              tunnel: [w876 w877] -> w871
              tunnel: w870 -> [w876 _]
              frame False {
              }
              frame True {
                n530 = property on="nPlotPerRun" class="DigNum (strict)"() -> ("Value"=w877:u64)  [unwired: 2 in, 2 out]
              }
            }
            n531 = Bundle("Averaging"=w874, "weighting mode"=w870, "Value"=w871) -> (w873:T10)  [unwired: 1 in]
            n532 = property on="Averaging" class="Clust (strict)"("Value"=w873) -> ()  [unwired: 2 in, 2 out]
          }
          event "Manual Save": Mouse Down; "Write Light": Value Change {
            n533 = event-data() -> ()  [unwired: 3 out]
            n534 = flat-sequence {
              frame #0 {
                n535 = local write "stop"(FALSE) -> ()
                "Location" <- "Start of \"Save\""
              }
              frame #1 {
                w893 = 10.0
                w894 = -10.0
                w891 = "MultiQ Data File:\\t%s \\n\\nSample Name:\\t%s \\nSample Label:\\t %s\\nDate:\\t%s \\nTime:\\t %s \\nWho:\\t%s \\nRun Number:\\t%d \\nDuration:\\t %.6f s \\nRate:\\t%7.2f Hz \\nData Points:\\t %d \\nRange:\\t(%5.1f, %5.1f) Volts\\nMin Frequency:\\t %9.2f kHz \\nPressure:\\t%9.2e torr\\nComment:\\t%s\\n\\n"  # MultiQ Data File:\t%s \n\nSample Name:\t%s \nSample Label:\t %s\nDate:\t%s \nTime:\t %s \nWho:\t%s \nRun Number:\t%d \nDuration:\t %.6f s \nRate:\t%7.2f Hz \nData Points:\t %d \nRange:\t(%5.1f, %5.1f) Volts\nMin Frequency:\t %9.2f kHz \nPressure:\t%9.2e torr\nComment:\t%s\n\n
                # "Make the HTML Table"
                # "Make the Data File Header"
                # "Date"
                # "Time"
                # "Write HTML Data in Table Row"
                # "HTML File Exists?"
                # "Update the Run Number"
                n536 = property on="Start Time" class="AbsTime (strict)"() -> ("Value"=w917:timestamp)  [unwired: 2 in, 2 out]
                n537 = local read "NDataPointsOutput"() -> (w895:u64)
                n538 = local read "fSampleOutput"() -> (w896:dbl)
                n539 = local read "RunPeriod"() -> (w897:dbl)
                n540 = local read "Run Number"() -> (w890:i8)
                n541 = local read "Comment"() -> (w880:string)
                n542 = local read "fMinPlot"() -> (w899:dbl)
                n543 = Format Date/Time String(time format string (%c)="%d %b %Y", seconds (now)=w917) -> (date/time string=w913:string)  [unwired: 1 out]
                n544 = Format Date/Time String(time format string (%c)="%H:%M:%S", seconds (now)=w917) -> (date/time string=w912:string)  [unwired: 1 out]
                n545 = Number To Decimal String(number="Run Number", width (-)=2) -> (decimal integer string=w929:string)
                n546 = Path To String(path="Path") -> (string=w921:string)
                n547 = Strip Path(path="Path") -> (stripped path=w924:path, name=w898:string)
                n548 = call <vilib>:"Trim Whitespace.vi"("string"=w929) -> ("trimmed string"=w918:string)  [unwired: 1 in]
                n549 = Format Into String(format string="<h2><b>Sample: </b>#%s,  %s </h2>", "Name", "Label") -> (resulting string=→"HTML \nTitle":string)  [unwired: 2 in, 1 out]
                n550 = Concatenate Strings(w898, "_", w918, ".txt") -> (w883:string)
                n551 = Concatenate Strings(w921, "_table.html") -> (w926:string)
                n552 = Build Path(base path=w924, name or relative path=w883) -> (appended path=w886:path)
                n553 = String To Path(string=w926) -> (path=w916:path)
                n554 = Format Into String(format string=w891, w883, "Name", "Label", w913, w912, "Who", w890, w897, w896, w895, w894, w893, w899, "Pressure (t)", w880) -> (resulting string=w905:string, error out=w906:errorcluster)  [unwired: 2 in]
                n555 = Format Into String(format string="<tr  align=\"center\" valign=\"middle\"> \\n <td>%s</td> <td>%s</td>  <td>%s</td> <td>%d</td>\n<td>%.6f</td> <td>%7.2f </td>\n<td>%d</td> <td>%5.1f</td>\n<td>%5.1f</td> <td>%9.2f</td> \n<td>%9.2e</td>\n<td>%s</td> <td>%s</td>\\n \n</tr>\\n\\n", error in=w906, w913, w912, "Who", w890, w897, w896, w895, w894, w893, w899, "Pressure (t)", w883, w880) -> (resulting string=w904:string, error out=w903:errorcluster)  [unwired: 1 in]
                n556 = local read "DataFilePath"() -> (w887:path)
                n557 = Equal?(x=w887, y=w886) -> (x = y?=w888:bool)
                n558 = local read "WriteNewHeader"() -> (w884:bool)
                n559 = case shown="False" w888 {
                  tunnel: w887 -> [w954 w955]
                  tunnel: w886 -> [w953 _]
                  tunnel: [w952 w955] -> w885
                  frame False {
                    n560 = Move(source path=w954, 10:w953) -> (3:w952:path)  [unwired: 3 in, 2 out]
                  }
                  frame True {
                  }
                }
                n561 = case shown="True" w884 {
                  tunnel: w905 -> [_ w946]
                  tunnel: w903 -> [w940 w945]
                  tunnel: [w940 w944] -> w902
                  tunnel: [w939 w943] -> w901
                  tunnel: w885 -> [w939 w941]
                  frame False {
                  }
                  frame True {
                    # "Open the Data File\nWrite Header"
                    n562 = Open/Create/Replace File(file path (use dialog)=w941, error in=w945, operation (0:open)=T5."open", access (0:read/write)=enum16{"read/write", "read-only", "write-only"}."write-only") -> (refnum out=w950:refnum<file>, error out=w949:errorcluster)  [unwired: 3 out]
                    n563 = Write to Text File(file (use dialog)=w950, text=w946, error in=w949) -> (refnum out=w942:refnum<file>, error out=w947:errorcluster)  [unwired: 2 out]
                    n564 = Close File(refnum=w942, error in=w947) -> (path=w943:path, error out=w944:errorcluster)
                  }
                }
                n565 = call <vilib>:"Check if File or Folder Exists.vi"("error in (no error)"=w902, "path"=w916) -> ("error out"=w933:errorcluster, "file or folder exists?"=w935:bool, "dup path"=w934:path)  [unwired: 7 out]
                n566 = case shown="False" w935 {
                  tunnel: w934 -> [w964 w971]
                  tunnel: w933 -> [w965 w970]
                  tunnel: [w961 w969] -> w932
                  tunnel: [w959 w968] -> w931
                  frame False {
                    # "Create File & Write Header Row"
                    n567 = Open/Create/Replace File(file path (use dialog)=w964, error in=w965, operation (0:open)=T5."create", access (0:read/write)=enum16{"read/write", "read-only", "write-only"}."write-only") -> (refnum out=w963:refnum<file>, error out=w962:errorcluster)  [unwired: 3 out]
                    n568 = property on="HTML \nTitle" class="Str"() -> ("Value"=w957:string)  [unwired: 2 in, 2 out]
                    n569 = Format Into String(format string="%s\\n%s\\n%s\\n\\n", initial string=w963, error in=w962, w957, "<table border=\"1\" cellspacing =\"1\" cellpadding=\"6\">", "<tr  align=\"center\" valign=\"middle\"> <th>Date</th> <th>Time</th> <th>Who</th><th>Run #</th> <th>Duration (s)</th> <th>Rate (Hz)</th> <th>N Points</th> <th>Min Value (V)</th> <th>Max Value (V)</th><th>Min Freq (jkHz)</th> <th>Pressure (torr)</th>  <th>Filename</th><th>Comment</th> </tr>") -> (resulting string=w961:refnum<file>, error out=w959:errorcluster)
                  }
                  frame True {
                    # "Open File and Go To End"
                    n570 = Open/Create/Replace File(file path (use dialog)=w971, error in=w970, operation (0:open)=T5."open", access (0:read/write)=enum16{"read/write", "read-only", "write-only"}."write-only") -> (refnum out=w975:refnum<file>, error out=w974:errorcluster)  [unwired: 3 out]
                    n571 = Set File Position(refnum=w975, from (0:start)=1, error in=w974) -> (refnum out=w969:refnum<file>, error out=w968:errorcluster)  [unwired: 1 out]
                  }
                }
                n572 = Write to Text File(file (use dialog)=w932, text=w904, error in=w931) -> (refnum out=w938:refnum<file>, error out=w937:errorcluster)  [unwired: 2 out]
                n573 = Close File(refnum=w938, error in=w937) -> (error out=w936:errorcluster)  [unwired: 1 out]
                n574 = call <vilib>:"Simple Error Handler.vi"("type of dialog (OK msg:1)"=3, "error in (no error)"=w936) -> ("error?"=w881:bool)  [unwired: 7 out]
                n575 = case shown="False" w881 {
                  tunnel: w901 -> [w980 _]
                  tunnel: [w980 path ""] -> w914
                  tunnel: [2 0] -> w882
                  frame False {
                    n576 = property on="Run Number" class="DigNum (strict)"() -> ("Value"=w977:i8)  [unwired: 2 in, 2 out]
                    n577 = Increment(x=w977) -> (x+1=w979:i8)
                    n578 = property on="Run Number" class="DigNum (strict)"("Val(Sgnl)"=w979) -> ()  [unwired: 2 in, 2 out]
                  }
                  frame True {
                  }
                }
                "Out" <- w914
                n579 = property on="Manual Save" class="Bool (strict)"("Val(Sgnl)"=w881) -> ()  [unwired: 2 in, 2 out]
                n580 = property on="Write Light" class="Bool (strict)"("Value"=w881) -> ()  [unwired: 2 in, 2 out]
                n581 = property on="Manual Save" class="Bool (strict)"("DisabledEnum"=w882) -> ()  [unwired: 2 in, 2 out]
                n582 = Strip Path(path=w914) -> (name=→"File":string)  [unwired: 1 out]
              }
              frame #2 {
                n583 = local write "Location"("End of \"Save\"") -> ()
              }
            }
          }
          event "Substrate", "Mode Scale", "Range (%)", "Sample Modes": Value Change {
            w987 = 3
            w1004 = 7
            w1006 = 6
            w1020 = 1
            w1014 = 2
            w1012 = 3
            w1010 = 4
            w1008 = 5
            w1016 = 0
            # "1100 - 1150,  1750-1800,  2250-2600, 3975--4025,  4400--4500,  6175--6275"
            n584 = event-data() -> ()  [unwired: 7 out]
            n585 = case shown="0, Default" "Substrate" {
              tunnel: [dbl[] [328.16, 495.4, 753.66, 1157.4, 1313.3, 2003.9, 2014.8, 2175.7, 2822.6, 3043.4, 3398.1, 3767.8, 4232.0, 4806.5, 4837.8, 4986.6, 5573.5, 6031.7, 6389.6, 6767.0, 7063.3, 7348.2, 8139.4, 8697.8, 8729.1, 8786.8, 8920.1, 10050.0, 10347.0] dbl[] [1092.3, 1649.9, 2505.8, 3847.7, 4361.2, 6645.1, 6683.3, 7225.3, 9346.1, 10072.0, 11259.0, 12454.0, 13972.0, 15881.0, 15961.0, 16483.0, 18354.0, 19859.0, 21048.0, 22299.0, 23198.0, 24139.0, 26725.0, 28486.0, 28665.0, 28795.0, 29295.0, 32885.0, 33819.0] dbl[] [2760.1, 4168.9, 6298.4, 9640.0, 10894.0, 16481.0, 16575.0, 17940.0, 22992.0, 24705.0, 27613.0, 30365.0, 33870.0, 37411.0, 38418.0, 38537.0, 39856.0, 41993.0, 43948.0, 47449.0, 48423.0, 50180.0, 53083.0, 54835.0, 57044.0, 57205.0, 62763.0, 64874.0, 66442.0]] -> w984
              tunnel: [0.1 0.5 2.0] -> w1026
              tunnel: [11.0 35.0 70.0] -> w1025
              tunnel: [u8[] [1, 3, 5, 6, 9, 12, 15, 18, 22, 26, 29] u8[] [1, 3, 5, 6, 9, 12, 15, 18, 22, 26, 29] u8[] [1, 3, 5, 6, 9, 12, 16, 20, 25, 0, 0]] -> w996
              tunnel: [u8[] [1, 3, 4, 5, 6, 7, 9, 10, 11, 12, 13, 14, 15, 17, 18, 19, 20, 21, 22, 23, 24, 25, 26, 28, 29] u8[] [1, 3, 4, 5, 6, 7, 9, 10, 11, 12, 13, 14, 15, 17, 18, 19, 20, 21, 22, 23, 24, 25, 26, 28, 29] u8[] [1, 3, 4, 5, 6, 7, 9, 10, 11, 12, 13, 14, 15, 16, 19, 20, 21, 22, 23, 24, 25, 26, 27, 28, 29]] -> w985
              frame 0, Default {
              }
              frame 1 {
              }
              frame 2 {
              }
            }
            "All Modes" <- w984
            n586 = property on="fMaxPlot" class="DigNum (strict)"("Val(Sgnl)"=w1025) -> ()  [unwired: 2 in, 2 out]
            n587 = property on="fMinPlot" class="DigNum (strict)"("Val(Sgnl)"=w1026) -> ()  [unwired: 2 in, 2 out]
            n588 = for {
              tunnel: w985 -> [w1052] mode=indexing
              tunnel: w984 -> [w1053]
              tunnel: [w1051] -> w986 mode=indexing
              n589 = Index Array(array=w1053, index=w1052) -> (element=w1051:dbl)
            }
            "Nodal Modes" <- w986
            n590 = for {
              tunnel: w996 -> [w1055] mode=indexing
              tunnel: w984 -> [w1056]
              tunnel: [w1054] -> w988 mode=indexing
              n591 = Index Array(array=w1056, index=w1055) -> (element=w1054:dbl)
            }
            "Shear Modes" <- w988
            n592 = for {
              N: 2 -> [_]
              tunnel: w996 -> [w1061]
              tunnel: [w1057] -> w991 mode=indexing
              tunnel: [w1058] -> w995 mode=indexing
              tunnel: w984 -> [w1060]
              i -> [w1059]
              n593 = for {
                N: 8 -> [_]
                tunnel: [w1069] -> w1058 mode=indexing
                tunnel: w1059 -> [w1068]
                tunnel: w1061 -> [w1067] mode=indexing
                tunnel: w1060 -> [w1064]
                tunnel: [w1063] -> w1057 mode=indexing
                i -> [w1066]
                n594 = case shown="0, Default" w1068 {
                  tunnel: [w1078 w1080] -> w1065
                  tunnel: w1067 -> [_ w1080]
                  tunnel: w1066 -> [w1076 _]
                  tunnel: w1064 -> [w1077 w1082]
                  tunnel: [w1075 w1079] -> w1063
                  frame 0, Default {
                    n595 = Increment(x=w1076) -> (x+1=w1078:i32)
                    n596 = Index Array(array=w1077, index=w1076) -> (element=w1075:dbl)
                  }
                  frame 1 {
                    n597 = Decrement(x=w1080) -> (x-1=w1081:u8)
                    n598 = Index Array(array=w1082, index=w1081) -> (element=w1079:dbl)
                  }
                }
                n599 = Number To Decimal String(number=w1065) -> (decimal integer string=w1073:string)  [unwired: 1 in]
                n600 = Number To Decimal String(number=w1063) -> (decimal integer string=w1071:string)  [unwired: 1 in]
                n601 = Concatenate Strings("Mode ", w1073, ": ", w1071, " Hz (FEM)") -> (w1069:string)
              }
            }
            "PlotLabelArray" <- w995
            "PlotFreqArray" <- w991
            n602 = Array Subset(array=w984, index=0, length=w987) -> (→"Modes 1-3":dbl[])
            n603 = Array Subset(array=w984, index=3, length=w987) -> (→"Modes 4-6":dbl[])
            n604 = Array Subset(array=w984, index=6, length=w987) -> (→"Modes 7-9":dbl[])
            n605 = Array Subset(array=w984, index=9, length=w987) -> (→"Modes 10-12":dbl[])
            n606 = Array Size(array=w995) -> (size(s)=→"PlotLabelSize":i32[])
            n607 = Array Size(array=w991) -> (size(s)=→"PlotModeSize":i32[])
            n608 = Index Array(array=w991, index (row)="Sample Modes") -> (element=w989:dbl[])  [unwired: 1 in]
            n609 = Index Array(array=w995, index (row)="Sample Modes") -> (element=w992:string[])  [unwired: 1 in]
            n610 = Divide(x="Range (%)", y=100.0) -> (x/y=w1047:dbl)
            n611 = Multiply(x="Mode Scale", y=w989) -> (x*y=w1018:dbl[])
            n612 = Increment(x=w1047) -> (x+1=w1017:dbl)
            n613 = Subtract(x=1.0, y=w1047) -> (x-y=w1046:dbl)
            n614 = Multiply(x=w1018, y=w1046) -> (x*y=w1045:dbl[])
            n615 = Multiply(x=w1018, y=w1017) -> (x*y=w1036:dbl[])
            n616 = Index Array(array=w992, index=w1016) -> (element=→"Plot1Label":string)
            n617 = Index Array(array=w1036, index=w1016) -> (element=w1035:dbl)
            n618 = Index Array(array=w1045, index=w1016) -> (element=w1044:dbl)
            n619 = property on="Plot1" class="WFGraph (strict)"("XScale.Maximum"=w1035) -> ()  [unwired: 2 in, 2 out]
            n620 = property on="Plot1" class="WFGraph (strict)"("XScale.Minimum"=w1044) -> ()  [unwired: 2 in, 2 out]
            n621 = Index Array(array=w992, index=w1020) -> (element=→"Plot2Label":string)
            n622 = Index Array(array=w1045, index=w1020) -> (element=w1043:dbl)
            n623 = Index Array(array=w1036, index=w1020) -> (element=w1034:dbl)
            n624 = property on="Plot2" class="WFGraph (strict)"("XScale.Minimum"=w1043) -> ()  [unwired: 2 in, 2 out]
            n625 = property on="Plot2" class="WFGraph (strict)"("XScale.Maximum"=w1034) -> ()  [unwired: 2 in, 2 out]
            n626 = Index Array(array=w992, index=w1014) -> (element=→"Plot3Label":string)
            n627 = Index Array(array=w1045, index=w1014) -> (element=w1042:dbl)
            n628 = Index Array(array=w1036, index=w1014) -> (element=w1033:dbl)
            n629 = property on="Plot3" class="WFGraph (strict)"("XScale.Minimum"=w1042) -> ()  [unwired: 2 in, 2 out]
            n630 = property on="Plot3" class="WFGraph (strict)"("XScale.Maximum"=w1033) -> ()  [unwired: 2 in, 2 out]
            n631 = Index Array(array=w992, index=w1012) -> (element=→"Plot4Label":string)
            n632 = Index Array(array=w1036, index=w1012) -> (element=w1032:dbl)
            n633 = Index Array(array=w1045, index=w1012) -> (element=w1041:dbl)
            n634 = property on="Plot4" class="WFGraph (strict)"("XScale.Maximum"=w1032) -> ()  [unwired: 2 in, 2 out]
            n635 = property on="Plot4" class="WFGraph (strict)"("XScale.Minimum"=w1041) -> ()  [unwired: 2 in, 2 out]
            n636 = Index Array(array=w992, index=w1010) -> (element=→"Plot5Label":string)
            n637 = Index Array(array=w1045, index=w1010) -> (element=w1040:dbl)
            n638 = Index Array(array=w1036, index=w1010) -> (element=w1031:dbl)
            n639 = property on="Plot5" class="WFGraph (strict)"("XScale.Minimum"=w1040) -> ()  [unwired: 2 in, 2 out]
            n640 = property on="Plot5" class="WFGraph (strict)"("XScale.Maximum"=w1031) -> ()  [unwired: 2 in, 2 out]
            n641 = Index Array(array=w992, index=w1008) -> (element=→"Plot6Label":string)
            n642 = Index Array(array=w1036, index=w1008) -> (element=w1030:dbl)
            n643 = Index Array(array=w1045, index=w1008) -> (element=w1039:dbl)
            n644 = property on="Plot6" class="WFGraph (strict)"("XScale.Minimum"=w1039) -> ()  [unwired: 2 in, 2 out]
            n645 = property on="Plot6" class="WFGraph (strict)"("XScale.Maximum"=w1030) -> ()  [unwired: 2 in, 2 out]
            n646 = Index Array(array=w992, index=w1006) -> (element=→"Plot7Label":string)
            n647 = Index Array(array=w1045, index=w1006) -> (element=w1038:dbl)
            n648 = Index Array(array=w1036, index=w1006) -> (element=w1029:dbl)
            n649 = property on="Plot7" class="WFGraph (strict)"("XScale.Minimum"=w1038) -> ()  [unwired: 2 in, 2 out]
            n650 = property on="Plot7" class="WFGraph (strict)"("XScale.Maximum"=w1029) -> ()  [unwired: 2 in, 2 out]
            n651 = Index Array(array=w992, index=w1004) -> (element=→"Plot8Label":string)
            n652 = Index Array(array=w1045, index=w1004) -> (element=w1037:dbl)
            n653 = Index Array(array=w1036, index=w1004) -> (element=w1028:dbl)
            n654 = property on="Plot8" class="WFGraph (strict)"("XScale.Minimum"=w1037) -> ()  [unwired: 2 in, 2 out]
            n655 = property on="Plot8" class="WFGraph (strict)"("XScale.Maximum"=w1028) -> ()  [unwired: 2 in, 2 out]
          }
          event "QUIT": Mouse Down {
            n656 = event-data() -> ()  [unwired: 4 out]
            n657 = call <vilib>:"Three Button Dialog.vi"("Window Title (\"\")"="Quit or Stop?", "Right Button Text (\"Cancel\")"="Cancel", "Center Button Text (\"No\")"="Stop", "Left Button Text (\"Yes\")"="Quit", "message"="Stop operation (debug) or Quit the applcation?") -> ("Which Button?"=w1100:T9)  [unwired: 6 out]
            n658 = case shown="\"Center Button\"" w1100 {
              tunnel: [TRUE TRUE FALSE FALSE] -> w1098
              frame "Left Button", Default {
              }
              frame "Center Button" {
              }
              frame "Right Button" {
              }
              frame "Window Close" {
              }
            }
            n659 = Greater Than 0?(x=w1100) -> (x > 0?=w1099:bool)
          }
          event "Unit", "Type": Value Change {
            n660 = event-data() -> ()  [unwired: 7 out]
            n661 = Equal To 0?(x="Type") -> (x = 0?=w1111:bool)
            n662 = Equal To 0?(x="Unit") -> (x = 0?=w1113:bool)
            n663 = case shown="False" w1113 {
              tunnel: [w1116 w1119] -> w1110
              tunnel: w1111 -> [w1115 w1120]
              frame False {
                n664 = case shown="False" w1115 {
                  tunnel: ["Power Density [Rad / rHz]" "Power [Rad]"] -> w1116
                  frame False {
                  }
                  frame True {
                  }
                }
              }
              frame True {
                n665 = case shown="True" w1120 {
                  tunnel: ["Power Density [V / V_total / rHz]" "Power [V / V_total]"] -> w1119
                  frame False {
                  }
                  frame True {
                  }
                }
              }
            }
            n666 = property on="Plot5" class="WFGraph (strict)"("YScale.NameLbl.Text"=w1110) -> ()  [unwired: 2 in, 2 out]
            n667 = property on="Plot6" class="WFGraph (strict)"("YScale.NameLbl.Text"=w1110) -> ()  [unwired: 2 in, 2 out]
            n668 = property on="Plot8" class="WFGraph (strict)"("YScale.NameLbl.Text"=w1110) -> ()  [unwired: 2 in, 2 out]
            n669 = property on="Plot7" class="WFGraph (strict)"("YScale.NameLbl.Text"=w1110) -> ()  [unwired: 2 in, 2 out]
            n670 = property on="Plot3" class="WFGraph (strict)"("YScale.NameLbl.Text"=w1110) -> ()  [unwired: 2 in, 2 out]
            n671 = property on="Plot4" class="WFGraph (strict)"("YScale.NameLbl.Text"=w1110) -> ()  [unwired: 2 in, 2 out]
            n672 = property on="Plot2" class="WFGraph (strict)"("YScale.NameLbl.Text"=w1110) -> ()  [unwired: 2 in, 2 out]
            n673 = property on="Plot1" class="WFGraph (strict)"("YScale.NameLbl.Text"=w1110) -> ()  [unwired: 2 in, 2 out]
            n674 = property on="PSD Y" class="WFGraph (strict)"("YScale.NameLbl.Text"=w1110) -> ()  [unwired: 2 in, 2 out]
            n675 = property on="PSD X" class="WFGraph (strict)"("YScale.NameLbl.Text"=w1110) -> ()  [unwired: 2 in, 2 out]
          }
        }
        n676 = Or(x=w23, y=w24) -> (x .or. y?=w22:bool)
      }
    }
    frame #2 {
      n677 = case shown="False" w1123 {
        frame False {
          n678 = Quit LabVIEW() -> ()  [unwired: 1 out]
        }
        frame True {
          n679 = Stop() -> ()  [unwired: 1 out]
        }
      }
    }
  }
